vi "Preference_Panel.vi"(0 "Mode":T1) -> ()   [LabVIEW 2010]
uses:
  Anemometry Sub Vis/Controls/Server_Comms.ctl
  Anemometry Sub Vis/Controls/Preference_Mode.ctl
  Anemometry Sub Vis/Controls/Overhead.ctl
  <vilib>/Instr/_visa.llb/VISA Find Search Mode.ctl
  ADAM Client/Sub VIs/ADAM Controls/Calib_type_ADAM.ctl
  ADAM Client/Sub VIs/ADAM Controls/Module_type_ADAM.ctl
  ADAM Client/Sub VIs/ADAM Controls/Ch_description_ADAM.ctl
  ADAM Client/Sub VIs/ADAM Controls/Function_ADAM.ctl
  ADAM Client/Sub VIs/ADAM Controls/Channel_State.ctl
  ADAM Client/Sub VIs/ADAM Controls/Address.ctl
  Anemometry Sub Vis/Globals/Constants_global.vi
  Anemometry Sub Vis/Globals/Preference_global.vi
  Anemometry Sub Vis/Globals/Trav_pos_global.vi
  Anemometry Sub Vis/Globals/Qnet_Globals.vi
  Anemometry Sub Vis/Acquisition/PWA/PWAtasksGLOBAL.vi
  Anemometry Sub Vis/Globals/Dynamic_call_global.ph.vi
panel:
  in  "Post Processing Machine":bool
  in  "Analogue Device Serial No.":string="1188AB4"
  in  "PWA Device Serial No.":string="1187C98"
  in  "ADAM Setup File":u16(ring) items=["Current_Setup.xls"]
  in  "Default Source Establishment Time (s)":dbl=20.0
  out "This Machine's IP Number":string
  in  "Rig Setup":u16(ring) items=["3_x_2_tunnel", "A_Tunnel", "Adam_Sayer_Desk", "ADAM_Server", "Aero_Tunnel", "Alex_Desktop", "B_Tunnel", "Calibration_Tunnel", "Contact_Conductance", "D_Tunnel", "EnFlo_Tunnel", "Frauke_Desktop", "iMac_G5_2", "iMacDuo1", "Matteo's_desktop", "Matteo_PC", "Nick_PC-2", "Paul_Desk-Paul_Desk_Machine", "Paul_Hayden-Desk", "Paul_N_Desk_Machine_2", "Post_Processing_Machine", "PowerBook_G4_1", "PowerBook_G4_2", "Syn_jet_rig", "Tank", "tdf", "Tom_Desk", "Towing_tank", "--New Rig Setup--"]
  in  "Default Traverse Name":u16(ring) items=["A_Tunnel", "Aero_ThroughWall", "Aero_Tunnel", "Angle_Calibrator", "B_Tunnel", "D_Tunnel", "Dummy_Traverse", "EnFlo_Stack", "EnFlo_Tunnel", "EnFlo_Turntable", "Laser_Meas_Traverse", "mohd_setup", "Paul_Desk_Test", "PIV_Traverse", "--New Traverse Setup--"]
  in  "OK":bool
  in  "% Error From First Calib":dbl=10.0 format="%.1f"
  in  "% Error From Previous Calib":dbl=0.5 format="%.1f"
  in  "Qnet Site Root":path=path "/G4_2_HD/Users/paulhayden/Qnet/qnet"
  out "Templates":path=path "/G4_2_HD/Applications (Mac OS 9)/EnFlo Software/Anemometry/Anemometry Sub Vis/Templates"
  in  "Data Folder":path
  out "EnFlo SW Preferences":path=path "/G4_2_HD/Applications (Mac OS 9)/LabVIEW 5.1/EnFlo SW Preferences"
  in  "Tunnel Speed Control":bool
  in  "SMTP server IP address":string
  in  "Abs Press (mbar)":string="Froude:NPL:Atmos_Press"
  in  "Temperature":string="EnFlo Tun:Inlet Heater:Av Temp"
  in  "Server port number":u32=3363
  in  "Server address":string
  in  "LabVIEW Administrators":string[](array[string])=["", "", "", "", "", "", "", "", "", "", "", "", "", "", "", "", "", "", "", ""]
  in  "Server Comms":T2=enum."Do Not Link To Server"
  # "Server Computer Peferences"
  # "Multi Run Preferences"
  # "Warning Levels for Autocalibration Changes"
  # "Email Peferences"
  # "Deg C"
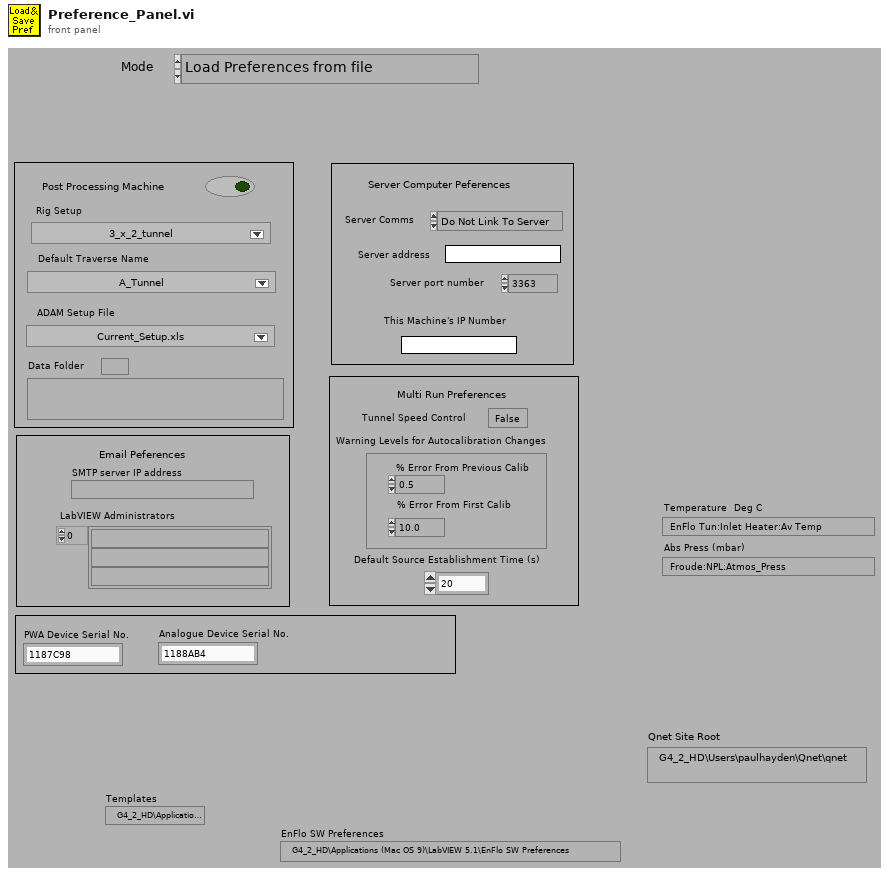
[diagram p1: front panel]
types:
  T1 = typedef "Preference_Mode.ctl" = enum16{"Load Preferences from file", "Save Preferences to file", "Load, Edit then Save"}
  T2 = typedef "Server_Comms.ctl" = enum16{"Server Link Healthy", "Do Not Link To Server"}
  T3 = enum8{"Enabled", "Disabled", "Disabled and Grayed Out"}
  T4 = typedef "Overhead.ctl" = enum16{"Update total times", "Read Current Overhead", "Re Scale totals to 3 hrs", "Initialise totals to 3hr"}
  T5 = typedef "Calib_type_ADAM.ctl" = enum16{"Raw", "Bx + A", "Cx^2 + Bx + A", "Dx^3 + Cx^2 + Bx + A", "In Band", "Hi-Tec Q", "Hi-Tec M_dot", "Text"}
  T6 = typedef "Module_type_ADAM.ctl" = enum16{"4011", "4012", "4013", "4014", "4016", "4017", "4018", "4021", "4050", "4052", "4053", "4060", "4080", "5000", "5017", "5018", "5024", "5051", "5056", "5060", "6060", "Tracker", "WEST", "GILL", "JEM", "VICI", "Vaisala", "DRUCK", "Run VI Named:", "IR2100", "PPT", "Comparator", "VIRTUAL", "Hold Value", "Read A", "Read Ch", "Coded", "Client Info", "Web Client", "X10", "Test"}
  T7 = typedef "Channel_State.ctl" = enum16{"On", "Off", "Always On", "Always Off"}
  T8 = typedef "VISA Find Search Mode.ctl" = u32
  T9 = typedef "Ch_description_ADAM.ctl" = cluster{"Ch Name":string, "Type":T6, "Function":T10, "Ch State":T7, "Calibration type":T5, "A":dbl, "B":dbl, "C":dbl, "D":dbl, "Comments":string, "Address":T11, "String":string, "Duty":u16}
  T10 = typedef "Function_ADAM.ctl" = enum16{"Analogue Input", "Digital Input", "Event counter", "Event rate", "Analogue Output", "Digital Output", "Relay Output"}
  T11 = typedef "Address.ctl" = cluster{"Main":i32, "Ch.":i32, "Sub":i32, "Port Name":string}
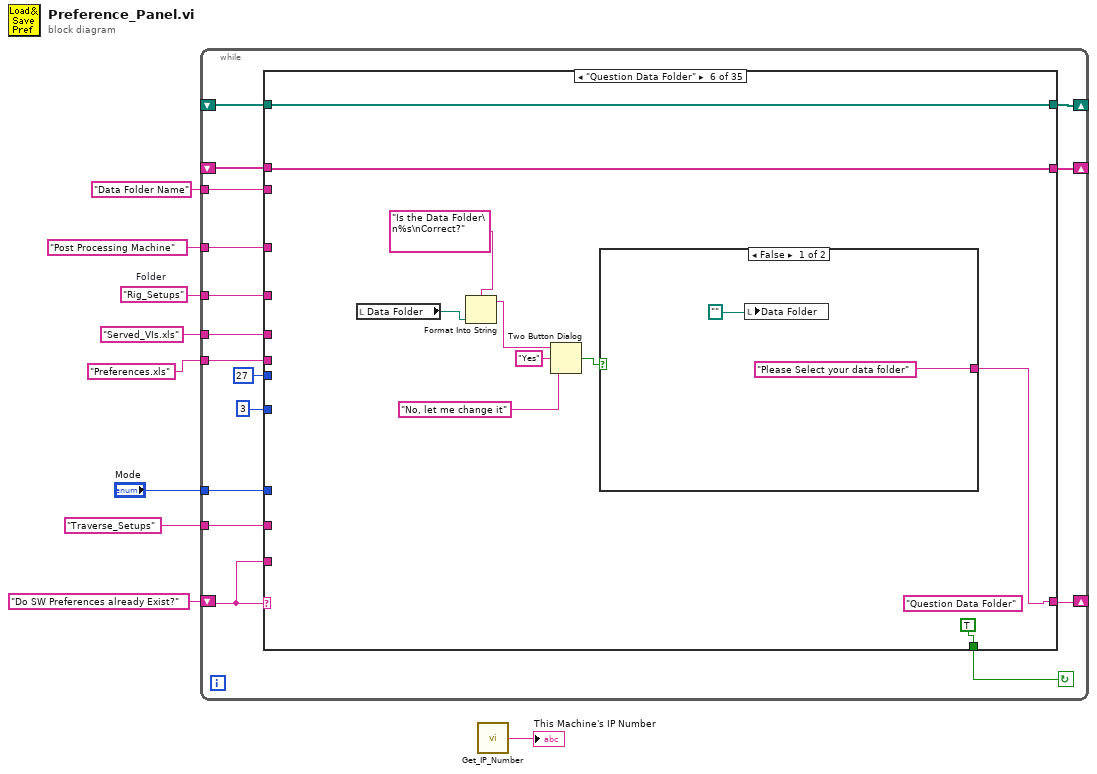
[diagram p0: block diagram]
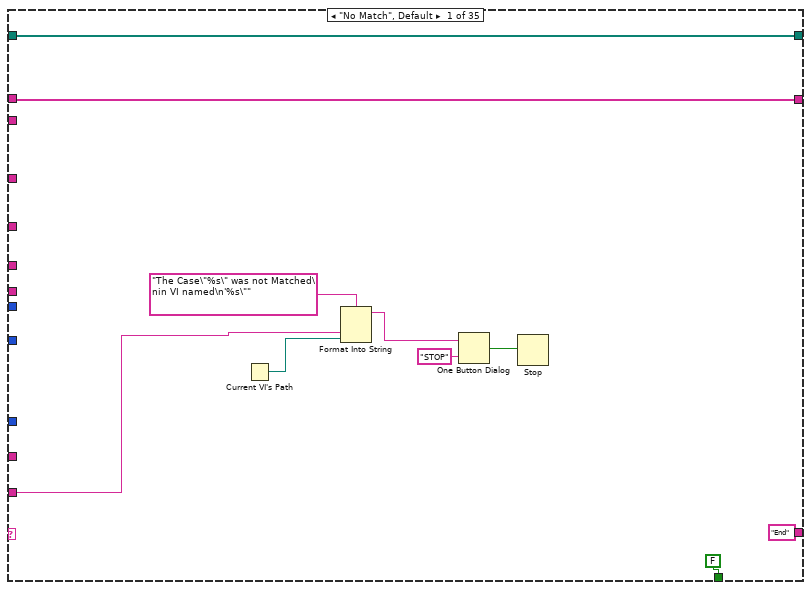
[diagram p2: hidden frame]
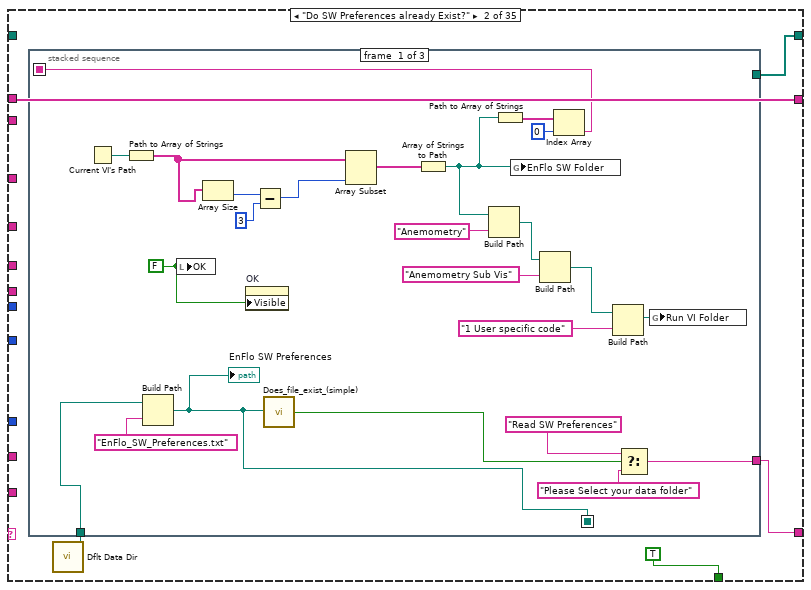
[diagram p3: hidden frame]
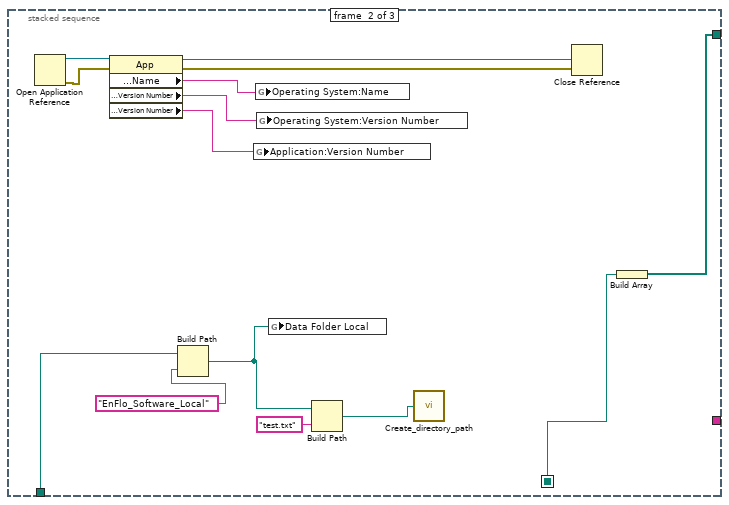
[diagram p4: hidden frame]
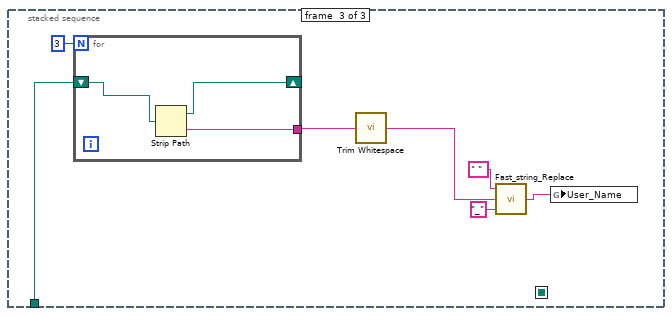
[diagram p5: hidden frame]
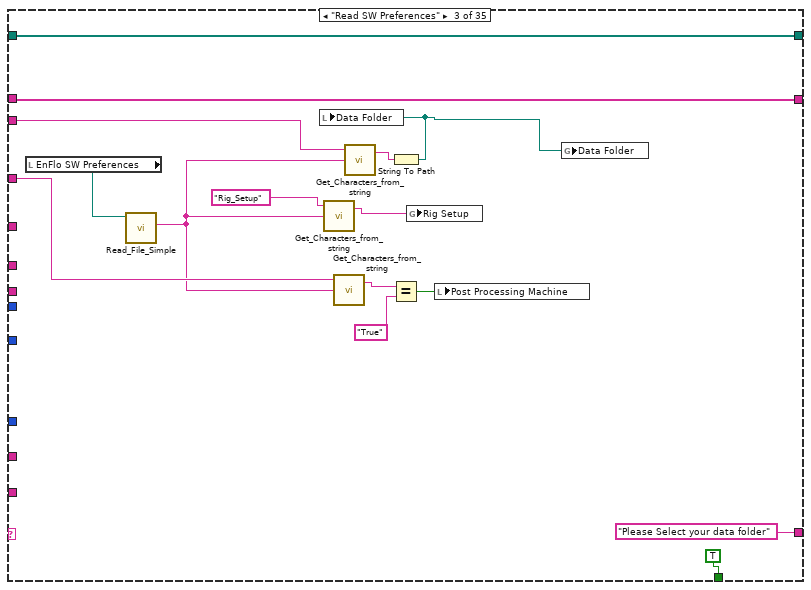
[diagram p6: hidden frame]
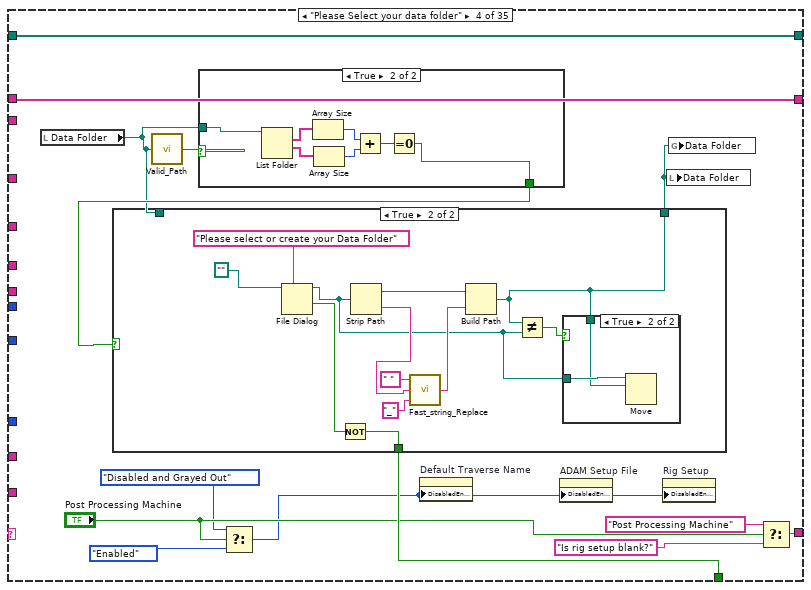
[diagram p7: hidden frame]
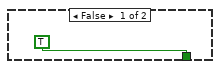
[diagram p8: hidden frame]
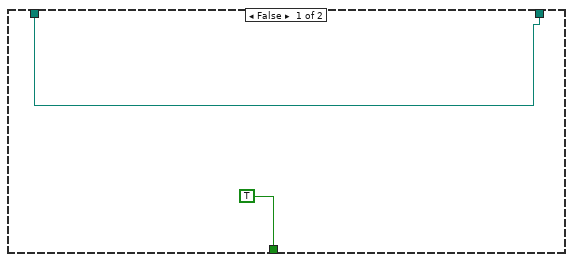
[diagram p9: hidden frame]
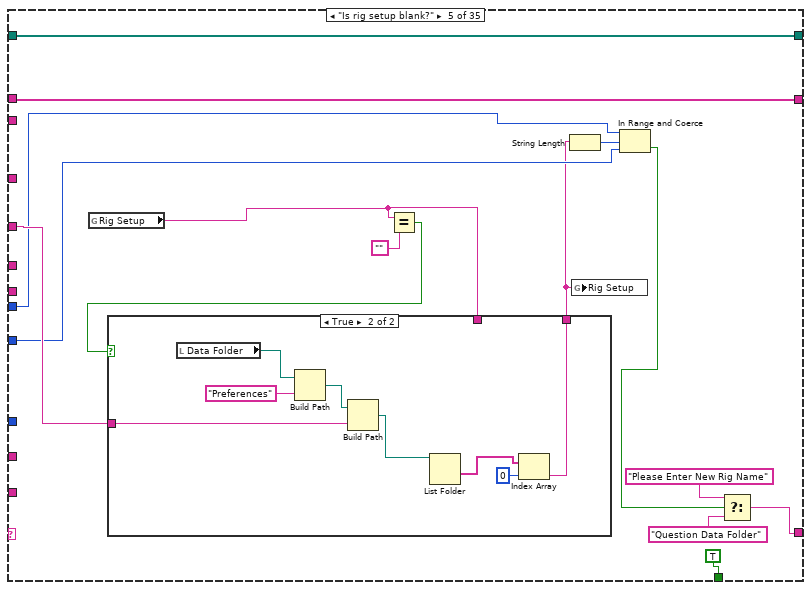
[diagram p11: hidden frame]
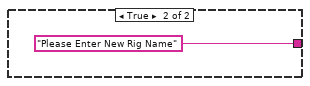
[diagram p13: hidden frame]
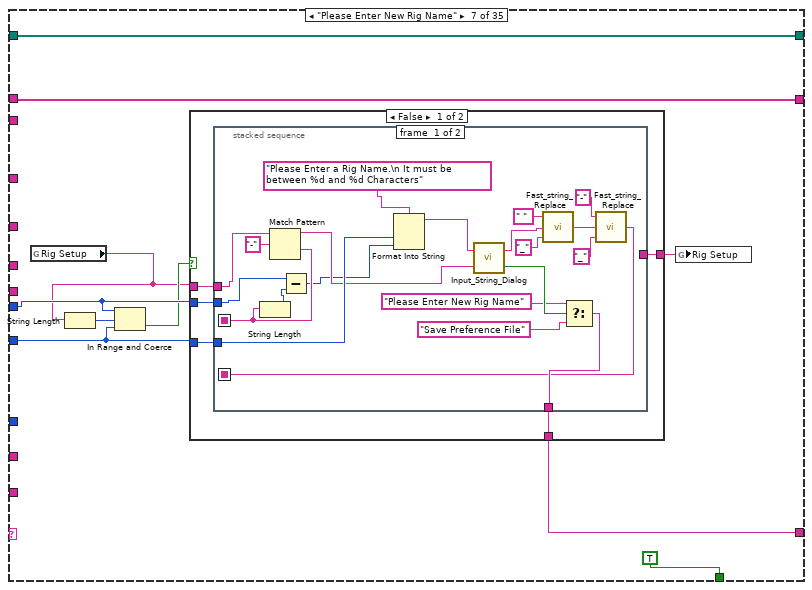
[diagram p14: hidden frame]
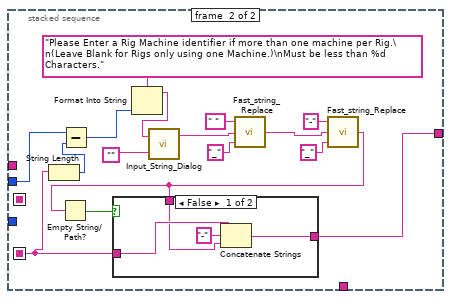
[diagram p15: hidden frame]
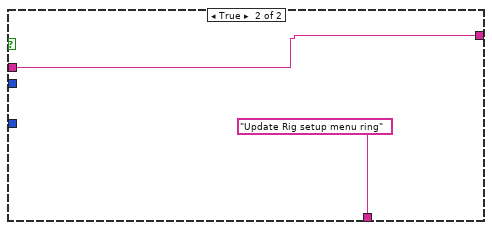
[diagram p17: hidden frame]
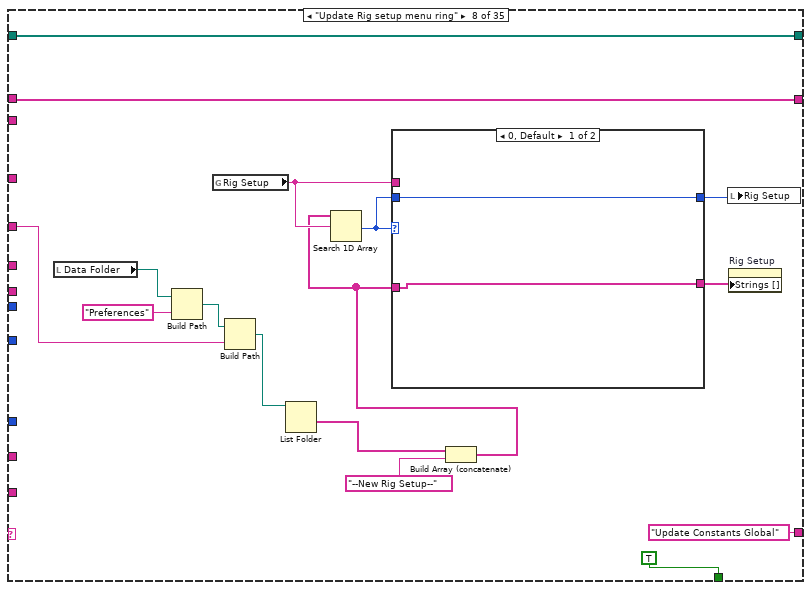
[diagram p18: hidden frame]
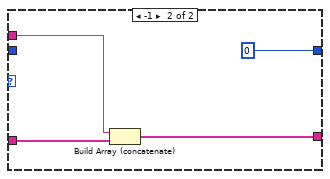
[diagram p19: hidden frame]
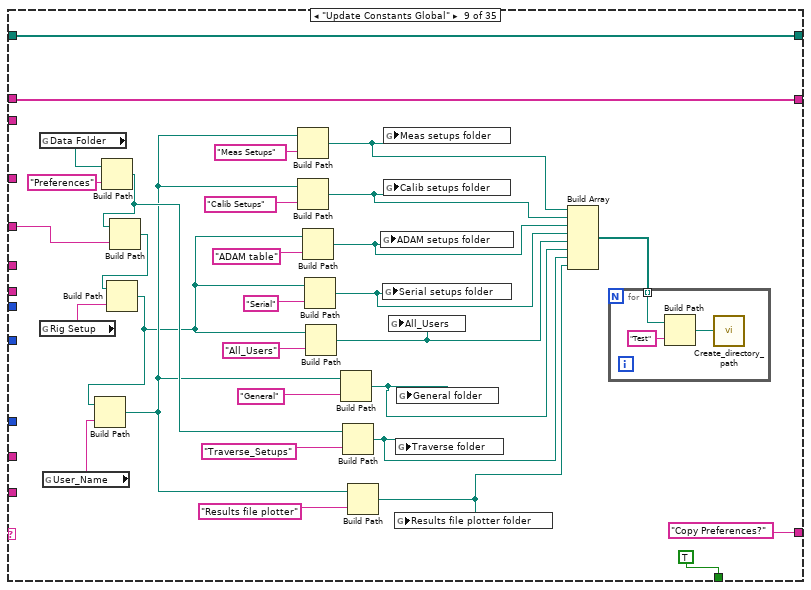
[diagram p20: hidden frame]
diagram:
  w4 = "Rig_Setups"  # Folder
  n1 = while {
    shift-left: _ -> [w22]
    shift-right: [w23] -> _
    shift-left: "Do SW Preferences already Exist?" -> [w21]
    shift-right: [w24] -> _
    tunnel: "Mode" -> [w20]
    tunnel: "Data Folder Name" ("Label for characters") -> [w19]
    tunnel: "Served_VIs.xls" ("Substring") -> [w18]
    tunnel: "Preferences.xls" ("name or relative path") -> [w17]
    tunnel: w4 -> [w14]
    tunnel: "Traverse_Setups" ("name or relative path") -> [w13]
    shift-right: [w12] -> _
    shift-left: _ -> [w11]
    tunnel: "Post Processing Machine" ("Label for characters") -> [w10]
    stop <- w25 continue-if-true
    n2 = case shown="\"Question Data Folder\"" w21 {
      tunnel: [FALSE TRUE TRUE w111 TRUE TRUE TRUE TRUE TRUE TRUE TRUE TRUE TRUE TRUE TRUE TRUE TRUE TRUE TRUE TRUE TRUE TRUE TRUE TRUE TRUE TRUE TRUE TRUE TRUE TRUE w867 TRUE TRUE TRUE FALSE] -> w25
      tunnel: ["End" w38 "Please Select your data folder" w108 w143 w166 w185 "Update Constants Global" ("f") "Copy Preferences?" "Copy Preferences?" w331 "Read SW Preferences" "Install Preference files" "Install Adam table files" "Install Adam setup files" "Choose ADAM Setup file" "Preference files continued" "Variable Names" w506 w523 "Please Enter new  Traverse Setup" w598 "Create Traverse setup" ("f") "Check file permission status" w694 w723 w743 w762 w779 "Save Preference File" "Save SW Preferences" w931 w944 "Initialise Globals" "End"] -> w24
      tunnel: [w27 w39 w102 w117 w155 w174 w187 w252 w288 w321 w329 w345 w392 w408 w433 w452 w474 w485 w511 w533 w586 w600 w634 w651 w695 w728 w748 w771 w784 w798 w873 w939 w945 w997 w1057] -> w23
      tunnel: w22 -> [w27 w39 w102 w117 w155 w174 w187 w252 w288 w321 w329 w345 w392 w408 w433 w452 w474 w485 _ w533 w586 w600 w634 w651 w695 w728 w748 w771 w784 w798 w873 w939 w945 w997 w1057]
      tunnel: w21 -> [w30 _ _ _ _ _ _ _ _ _ _ _ _ _ _ _ _ _ _ _ _ _ _ _ _ _ _ _ _ _ _ _ _ _ _]
      tunnel: w20 -> [_ _ _ _ _ _ _ _ _ _ _ _ _ _ _ _ _ _ w505 _ _ _ _ _ w693 _ _ _ _ _ w868 _ _ _ _]
      tunnel: w19 -> [_ _ w98 _ _ _ _ _ _ _ _ _ _ _ _ _ _ _ _ _ _ _ _ _ _ _ _ _ _ _ _ w930 _ _ _]
      tunnel: w18 -> [_ _ _ _ _ _ _ _ _ _ _ _ _ w402 _ _ _ _ _ _ _ _ _ _ _ _ _ _ _ _ _ _ _ w989 _]
      tunnel: w17 -> [_ _ _ _ _ _ _ _ _ _ w326 w343 _ _ _ _ _ _ _ w529 _ _ _ _ _ _ _ _ _ _ w865 _ _ _ _]
      tunnel: 3 ("lower limit") -> [_ _ _ _ w147 _ w184 _ _ _ _ _ _ _ _ _ _ _ _ _ _ w597 _ _ _ _ _ _ _ _ _ _ _ _ _]
      tunnel: 27 ("upper limit") -> [_ _ _ _ w148 _ w183 _ _ _ _ _ _ _ _ _ _ _ _ _ _ w596 _ _ _ _ _ _ _ _ _ _ _ _ _]
      tunnel: w14 -> [_ _ _ _ w152 _ _ w240 w268 w301 _ w342 _ _ _ _ _ _ _ _ _ _ _ _ _ _ _ _ _ _ _ _ _ _ _]
      tunnel: w13 -> [_ _ _ _ _ _ _ _ _ _ _ _ _ _ _ _ _ _ _ _ w584 _ w621 _ _ _ _ _ _ w797 _ _ _ _ _]
      tunnel: [w26 w36 w94 w112 w150 w173 w179 w238 w265 w300 w330 w346 w383 w398 w426 w449 w460 w476 w498 w527 w583 w592 w620 w647 path[] [] w720 w740 w765 w782 w796 w863 w927 w943 w988 w1054] -> w12
      tunnel: w11 -> [w26 _ w94 w112 w150 w173 w179 w238 w265 w300 w330 w346 w382 w400 w426 w450 w460 w478 w498 w528 w583 w592 w620 w648 w692 w720 w740 w765 w782 w796 w863 w927 w943 w988 w1054]
      tunnel: w10 -> [_ _ w93 _ _ _ _ _ _ _ _ _ _ _ _ _ _ _ _ _ _ _ _ _ _ _ _ _ _ _ _ w921 _ _ _]
      frame "No Match", Default {
        n3 = Current VI's Path() -> (path=w35:path)
        n4 = Format Into String(format string="The Case\"%s\" was not Matched\nin VI named\n'%s\"" ("Format String"), w30, w35) -> (resulting string=w32:string)  [unwired: 2 in, 1 out]
        n5 = One Button Dialog(message=w32, button name ("OK")="STOP") -> (true=w34:bool)
        n6 = Stop(stop? (T)=w34) -> ()
      }
      frame "Do SW Preferences already Exist?" {
        n7 = call <vilib>:"Dflt Data Dir.vi"() -> ("App:Default Data Directory"=w37:path)
        n8 = stacked-sequence {
          seq-local: [w44 _ _] -> [_ _ _]
          seq-local: [w42 _ _] -> [_ w70 _]
          tunnel: [w48 _ _] -> w38
          tunnel: w37 -> [w43 w68 w84]
          tunnel: [_ w71 _] -> w36
          frame #0 {
            w41 = FALSE ("OK")
            n9 = Current VI's Path() -> (path=w62:path)
            n10 = Path to Array of Strings(0:w62) -> (2:w59:string[])  [unwired: 1 out]
            n11 = Build Path(base path=w43, name or relative path="EnFlo_SW_Preferences.txt") -> (appended path=w42:path)
            "EnFlo SW Preferences" <- w42
            n12 = local write "OK"(w41) -> ()
            n13 = Array Size(array=w59) -> (size(s)=w61:i32)
            n14 = property on="OK" class="Bool (strict)"("Visible"=w41) -> ()  [unwired: 2 in, 2 out]
            n15 = Subtract(x=w61, y=3) -> (x-y=w57:i32)
            n16 = call "Does_file_exist_(simple).vi"("Pathname"=w42) -> ("exists?"=w63:bool)
            n17 = Array Subset(array=w59, length=w57) -> (w58:string[])  [unwired: 1 in]
            n18 = Array of Strings to Path(0:w58) -> (2:w45:path)  [unwired: 1 out]
            n19 = Build Path(base path=w45, name or relative path="Anemometry") -> (appended path=w54:path)
            n20 = Path to Array of Strings(0:w45) -> (2:w46:string[])  [unwired: 1 out]
            n21 = global write "Constants_global.vi" "EnFlo SW Folder"(w45) -> ()
            n22 = Build Path(base path=w54, name or relative path="Anemometry Sub Vis") -> (appended path=w52:path)
            n23 = Index Array(array=w46, index=0) -> (element=w44:string)
            n24 = Build Path(base path=w52, name or relative path="1 User specific code") -> (appended path=w51:path)
            n25 = Select(t="Read SW Preferences", s=w63, f="Please Select your data folder") -> (s? t:f=w48:string)
            n26 = global write "Constants_global.vi" "Run VI Folder"(w51) -> ()
          }
          frame #1 {
            n27 = Open Application Reference() -> (0:w75:errorcluster, 3:w78:refnum<vi>)  [unwired: 1 in, 3 out]
            n28 = property class="App"(reference=w78, error in=w75) -> (reference out=w77:refnum<vi>, error out=w76:errorcluster, "Operating System:Name"=w72:string, "Operating System:Version Number"=w74:string, "Application:Version Number"=w73:string)
            n29 = Build Path(base path=w68, name or relative path="EnFlo_Software_Local" ("element")) -> (appended path=w67:path)
            n30 = global write "Preference_global.vi" "Application:Version Number"(w73) -> ()
            n31 = global write "Preference_global.vi" "Operating System:Name"(w72) -> ()
            n32 = global write "Preference_global.vi" "Operating System:Version Number"(w74) -> ()
            n33 = global write "Constants_global.vi" "Data Folder Local"(w67) -> ()
            n34 = Build Path(base path=w67, name or relative path="test.txt") -> (appended path=w65:path)
            n35 = call "Create_directory_path.vi"("Path name"=w65) -> ()  [unwired: 1 out]
            n36 = Close Reference(reference=w77, error in (no error)=w76) -> ()  [unwired: 1 out]
            n37 = Build Array(w70) -> (w71:path[])
          }
          frame #2 {
            n38 = for {
              N: 3 -> [_]
              shift-right: [w88] -> _
              shift-left: w84 -> [w87]
              tunnel: [w86] -> w80
              n39 = Strip Path(path=w87) -> (stripped path=w88:path, name=w86:string)
            }
            n40 = call <vilib>:"Trim Whitespace.vi"("string"=w80) -> ("trimmed string"=w79:string)  [unwired: 1 in]
            n41 = call "Fast_string_Replace.vi"("Replace match with:"="_", "Input String"=w79, "regular expression"=" ") -> ("Output String"=w81:string)  [unwired: 1 in, 1 out]
            n42 = global write "Preference_global.vi" "User_Name"(w81) -> ()
          }
        }
      }
      frame "Read SW Preferences" {
        n43 = local read "EnFlo SW Preferences"() -> (w101:path)
        n44 = call "Read_File_Simple.vi"("Filename"=w101) -> ("string"=w92:string)  [unwired: 2 in, 7 out]
        n45 = call "Get_Characters_from_string.vi"("Input string"=w92, "Variable name"="Rig_Setup" ("Label for characters")) -> ("Value"=w95:string)  [unwired: 1 in, 1 out]
        n46 = call "Get_Characters_from_string.vi"("Input string"=w92, "Variable name"=w93) -> ("Value"=w91:string)  [unwired: 1 in, 1 out]
        n47 = call "Get_Characters_from_string.vi"("Input string"=w92, "Variable name"=w98) -> ("Value"=w99:string)  [unwired: 1 in, 1 out]
        n48 = String To Path(string=w99) -> (path=w97:path)
        n49 = local write "Data Folder"(w97) -> ()
        n50 = Equal?(x=w91, y="True") -> (x = y?=w89:bool)
        n51 = global write "Preference_global.vi" "Rig Setup"(w95) -> ()
        n52 = local write "Post Processing Machine"(w89) -> ()
        n53 = global write "Constants_global.vi" "Data Folder"(w97) -> ()
      }
      frame "Please Select your data folder" {
        n54 = local read "Data Folder"() -> (w113:path)
        n55 = call "Valid_Path.vi"("Filename"=w113) -> ("Valid Path?"=w115:bool)
        n56 = case shown="True" w115 {
          tunnel: [TRUE ("status") w119] -> w114
          tunnel: w113 -> [_ w125]
          frame False {
          }
          frame True {
            n57 = List Folder(path=w125) -> (filenames=w123:string[], folder names=w124:string[])  [unwired: 1 in, 4 out]
            n58 = Array Size(array=w123) -> (size(s)=w121:i32)
            n59 = Array Size(array=w124) -> (size(s)=w122:i32)
            n60 = Add(x=w121, y=w122) -> (x+y=w120:i32)
            n61 = Equal To 0?(x=w120) -> (x = 0?=w119:bool)
          }
        }
        n62 = case shown="True" w114 {
          tunnel: [w127 w130] -> w116
          tunnel: w113 -> [w127 _]
          tunnel: [TRUE w128] -> w111
          frame False {
          }
          frame True {
            n63 = File Dialog(7:"Please select or create your Data Folder" ("prompt"), 11:path "") -> (1:w129:bool, 3:w131:path)  [unwired: 1 in, 6 out]
            n64 = Not(x=w129) -> (.not. x?=w128:bool)
            n65 = Strip Path(path=w131) -> (stripped path=w135:path, name=w134:string)
            n66 = call "Fast_string_Replace.vi"("Replace match with:"="_", "Input String"=w134, "regular expression"=" ") -> ("Output String"=w133:string)  [unwired: 2 out]
            n67 = Build Path(base path=w135, name or relative path=w133) -> (appended path=w130:path)
            n68 = Not Equal?(x=w130, y=w131) -> (x != y?=w132:bool)
            n69 = case shown="True" w132 {
              tunnel: w131 -> [_ w141]
              tunnel: w130 -> [_ w140]
              frame False {
              }
              frame True {
                n70 = Move(source path=w141, 10:w140) -> ()  [unwired: 1 in, 5 out]
              }
            }
          }
        }
        n71 = Select(t=T3."Disabled and Grayed Out" ("Disabled"), s="Post Processing Machine", f=T3."Enabled" ("Disabled")) -> (s? t:f=w104:T3)
        n72 = property on="Default Traverse Name" class="Ring (strict)"("DisabledEnum"=w104) -> ()  [unwired: 2 in, 2 out]
        n73 = property on="ADAM Setup File" class="Ring (strict)"("DisabledEnum"=w104) -> ()  [unwired: 2 in, 2 out]
        n74 = property on="Rig Setup" class="Ring (strict)"("DisabledEnum"=w104) -> ()  [unwired: 2 in, 2 out]
        n75 = local write "Data Folder"(w116) -> ()
        n76 = global write "Constants_global.vi" "Data Folder"(w116) -> ()
        n77 = Select(t="Post Processing Machine", s="Post Processing Machine", f="Is rig setup blank?") -> (s? t:f=w108:string)
      }
      frame "Is rig setup blank?" {
        n78 = global read "Preference_global.vi" "Rig Setup"() -> (w151:string)
        n79 = Equal?(x=w151, y="") -> (x = y?=w153:bool)
        n80 = case shown="True" w153 {
          tunnel: w152 -> [_ w161]
          tunnel: [w157 w158] -> w146
          tunnel: w151 -> [w157 _]
          frame False {
          }
          frame True {
            n81 = local read "Data Folder"() -> (w164:path)
            n82 = Build Path(base path=w164, name or relative path="Preferences") -> (appended path=w163:path)
            n83 = Build Path(base path=w163, name or relative path=w161) -> (appended path=w162:path)
            n84 = List Folder(path=w162) -> (folder names=w159:string[])  [unwired: 1 in, 5 out]
            n85 = Index Array(array=w159, index=0) -> (element=w158:string)
          }
        }
        n86 = String Length(string=w146) -> (length=w149:i32)
        n87 = global write "Preference_global.vi" "Rig Setup"(w146) -> ()
        n88 = In Range and Coerce(upper limit=w148, x=w149, lower limit=w147) -> (In Range?=w145:bool)  [unwired: 1 out]
        n89 = Select(t="Please Enter New Rig Name", s=w145, f="Question Data Folder") -> (s? t:f=w143:string)
      }
      frame "Question Data Folder" {
        (unwired) "Question Data Folder"
        n90 = local read "Data Folder"() -> (w172:path)
        n91 = Format Into String(format string="Is the Data Folder\n%s\nCorrect?" ("message"), w172) -> (resulting string=w170:string)  [unwired: 2 in, 1 out]
        n92 = Two Button Dialog(message=w170, 1:"No, let me change it" ("F button name (\"Cancel\")"), 2:"Yes" ("T button name (\"OK\")")) -> (T button?=w167:bool)
        n93 = case shown="False" w167 {
          tunnel: ["Please Select your data folder" "Please Enter New Rig Name"] -> w166
          frame False {
            n94 = local write "Data Folder"(path "") -> ()
          }
          frame True {
          }
        }
      }
      frame "Please Enter New Rig Name" {
        n95 = global read "Preference_global.vi" "Rig Setup"() -> (w181:string)
        n96 = String Length(string=w181) -> (length=w186:i32)
        n97 = In Range and Coerce(upper limit=w183, x=w186, lower limit=w184) -> (In Range?=w182:bool)  [unwired: 1 out]
        n98 = case shown="False" w182 {
          tunnel: w181 -> [w193 w236]
          tunnel: [w189 "Update Rig setup menu ring"] -> w185
          tunnel: [w190 w236] -> w180
          tunnel: w184 -> [w192 _]
          tunnel: w183 -> [w191 _]
          frame False {
            n99 = stacked-sequence {
              seq-local: [w194 _] -> [_ w219]
              seq-local: [w201 _] -> [_ _]
              tunnel: w193 -> [w203 _]
              tunnel: w192 -> [w214 _]
              tunnel: w191 -> [w200 w217]
              tunnel: [_ w222] -> w190
              tunnel: [w206 _] -> w189
              frame #0 {
                n100 = Match Pattern(string=w203, regular expression="-") -> (before substring=w202:string, after substring=w201:string)  [unwired: 3 out]
                n101 = String Length(string=w201) -> (length=w199:i32)
                n102 = Subtract(x=w200, y=w199) -> (x-y=w198:i32)
                n103 = Format Into String(format string="Please Enter a Rig Name.\n It must be between %d and %d Characters" ("Message to user"), w214, w198) -> (resulting string=w213:string)  [unwired: 2 in, 1 out]
                n104 = call "Input_String_Dialog.vi"("Value"=w202, "Message to user"=w213) -> ("Ok Out"=w209:bool, "Output string"=w210:string)
                n105 = call "Fast_string_Replace.vi"("Replace match with:"="_", "Input String"=w210, "regular expression"=" ") -> ("Output String"=w195:string)  [unwired: 2 out]
                n106 = Select(t="Please Enter New Rig Name", s=w209, f="Save Preference File") -> (s? t:f=w206:string)
                n107 = call "Fast_string_Replace.vi"("Replace match with:"="_", "Input String"=w195, "regular expression"="-") -> ("Output String"=w194:string)  [unwired: 2 out]
              }
              frame #1 {
                n108 = String Length(string=w219) -> (length=w218:i32)
                n109 = Subtract(x=w217, y=w218) -> (x-y=w216:i32)
                n110 = Format Into String(format string="Please Enter a Rig Machine identifier if more than one machine per Rig.\n(Leave Blank for Rigs only using one Machine.)\nMust be less than %d Characters." ("Message to user"), w216) -> (resulting string=w215:string)  [unwired: 2 in, 1 out]
                n111 = call "Input_String_Dialog.vi"("Value"="", "Message to user"=w215) -> ("Output string"=w228:string)  [unwired: 1 out]
                n112 = call "Fast_string_Replace.vi"("Replace match with:"="_", "Input String"=w228, "regular expression"=" ") -> ("Output String"=w224:string)  [unwired: 2 out]
                n113 = call "Fast_string_Replace.vi"("Replace match with:"="_", "Input String"=w224, "regular expression"="-") -> ("Output String"=w221:string)  [unwired: 2 out]
                n114 = Empty String/Path?(string/path=w221) -> (empty?=w223:bool)
                n115 = case shown="False" w223 {
                  tunnel: [w231 w235] -> w222
                  tunnel: w219 -> [w234 w235]
                  tunnel: w221 -> [w232 _]
                  frame False {
                    n116 = Concatenate Strings(w234, "-" ("string"), w232) -> (w231:string)
                  }
                  frame True {
                  }
                }
              }
            }
          }
          frame True {
          }
        }
        n117 = global write "Preference_global.vi" "Rig Setup"(w180) -> ()
      }
      frame "Update Rig setup menu ring" {
        n118 = local read "Data Folder"() -> (w243:path)
        n119 = Build Path(base path=w243, name or relative path="Preferences") -> (appended path=w242:path)
        n120 = global read "Preference_global.vi" "Rig Setup"() -> (w249:string)
        n121 = Build Path(base path=w242, name or relative path=w240) -> (appended path=w241:path)
        n122 = List Folder(path=w241) -> (folder names=w239:string[])  [unwired: 1 in, 5 out]
        n123 = Build Array (concatenate)(w239, "--New Rig Setup--") -> (w245:string[])
        n124 = Search 1D Array(1D array=w245, element=w249) -> (index of element=w248:i32)  [unwired: 1 out]
        n125 = case shown="0, Default" w248 {
          tunnel: [w255 0] -> w251
          tunnel: w245 -> [w254 w258]
          tunnel: w249 -> [_ w257]
          tunnel: w248 -> [w255 _]
          tunnel: [w254 w256] -> w247
          frame 0, Default {
          }
          frame -1 {
            n126 = Build Array (concatenate)(w257, w258) -> (w256:string[])
          }
        }
        n127 = local write "Rig Setup"(w251) -> ()
        n128 = property on="Rig Setup" class="Ring (strict)"("Strings []"=w247) -> ()  [unwired: 2 in, 2 out]
      }
      frame "Update Constants Global" {
        n129 = global read "Constants_global.vi" "Data Folder"() -> (w266:path)
        n130 = global read "Preference_global.vi" "Rig Setup"() -> (w267:string)
        n131 = global read "Preference_global.vi" "User_Name"() -> (w264:string)
        n132 = Build Path(base path=w266, name or relative path="Preferences") -> (appended path=w269:path)
        n133 = Build Path(base path=w269, name or relative path=w268) -> (appended path=w270:path)
        n134 = Build Path(base path=w270, name or relative path=w267) -> (appended path=w260:path)
        n135 = Build Path(base path=w260, name or relative path=w264) -> (appended path=w263:path)
        n136 = Build Path(base path=w263, name or relative path="Meas Setups") -> (appended path=w280:path)
        n137 = Build Path(base path=w263, name or relative path="Calib Setups") -> (appended path=w279:path)
        n138 = Build Path(base path=w260, name or relative path="ADAM table") -> (appended path=w278:path)
        n139 = Build Path(base path=w260, name or relative path="Serial") -> (appended path=w277:path)
        n140 = Build Path(base path=w260, name or relative path="All_Users") -> (appended path=w261:path)
        n141 = Build Path(base path=w263, name or relative path="General") -> (appended path=w276:path)
        n142 = Build Path(base path=w269, name or relative path="Traverse_Setups") -> (appended path=w275:path)
        n143 = Build Path(base path=w263, name or relative path="Results file plotter") -> (appended path=w271:path)
        n144 = global write "Constants_global.vi" "ADAM setups folder"(w278) -> ()
        n145 = global write "Constants_global.vi" "Serial setups folder"(w277) -> ()
        n146 = global write "Constants_global.vi" "Meas setups folder"(w280) -> ()
        n147 = global write "Constants_global.vi" "Calib setups folder"(w279) -> ()
        n148 = global write "Constants_global.vi" "All_Users"(w261) -> ()
        n149 = global write "Constants_global.vi" "Results file plotter folder"(w271) -> ()
        n150 = global write "Constants_global.vi" "Traverse folder"(w275) -> ()
        n151 = global write "Constants_global.vi" "General folder"(w276) -> ()
        n152 = Build Array(w280, w279, w278, w277, w261, w276, w275, w271) -> (w274:path[])
        n153 = for {
          tunnel: w274 -> [w292] mode=indexing
          n154 = Build Path(base path=w292, name or relative path="Test") -> (appended path=w290:path)
          n155 = call "Create_directory_path.vi"("Path name"=w290) -> ()  [unwired: 1 out]
        }
      }
      frame "Post Processing Machine" {
        w298 = "Post_Processing_Machine" ("Rig Setup")
        n156 = global read "Constants_global.vi" "Data Folder Local"() -> (w299:path)
        n157 = global read "Preference_global.vi" "User_Name"() -> (w297:string)
        n158 = global write "Preference_global.vi" "Rig Setup"(w298) -> ()
        n159 = Build Path(base path=w299, name or relative path="Preferences") -> (appended path=w302:path)
        n160 = Build Path(base path=w302, name or relative path=w301) -> (appended path=w303:path)
        n161 = Build Path(base path=w303, name or relative path=w298) -> (appended path=w293:path)
        n162 = Build Path(base path=w293, name or relative path=w297) -> (appended path=w296:path)
        n163 = Build Path(base path=w296, name or relative path="Meas Setups") -> (appended path=w313:path)
        n164 = Build Path(base path=w296, name or relative path="Calib Setups") -> (appended path=w312:path)
        n165 = Build Path(base path=w293, name or relative path="ADAM table") -> (appended path=w311:path)
        n166 = Build Path(base path=w293, name or relative path="Serial") -> (appended path=w310:path)
        n167 = Build Path(base path=w293, name or relative path="All_Users") -> (appended path=w294:path)
        n168 = Build Path(base path=w296, name or relative path="General") -> (appended path=w309:path)
        n169 = Build Path(base path=w302, name or relative path="Traverse_Setups") -> (appended path=w308:path)
        n170 = Build Path(base path=w296, name or relative path="Results file plotter") -> (appended path=w304:path)
        n171 = global write "Constants_global.vi" "ADAM setups folder"(w311) -> ()
        n172 = global write "Constants_global.vi" "Serial setups folder"(w310) -> ()
        n173 = global write "Constants_global.vi" "Meas setups folder"(w313) -> ()
        n174 = global write "Constants_global.vi" "Calib setups folder"(w312) -> ()
        n175 = global write "Constants_global.vi" "All_Users"(w294) -> ()
        n176 = global write "Constants_global.vi" "Results file plotter folder"(w304) -> ()
        n177 = global write "Constants_global.vi" "Traverse folder"(w308) -> ()
        n178 = global write "Constants_global.vi" "General folder"(w309) -> ()
        n179 = Build Array(w313, w312, w311, w310, w294, w309, w308, w304) -> (w307:path[])
        n180 = for {
          tunnel: w307 -> [w325] mode=indexing
          n181 = Build Path(base path=w325, name or relative path="Test") -> (appended path=w323:path)
          n182 = call "Create_directory_path.vi"("Path name"=w323) -> ()  [unwired: 1 out]
        }
      }
      frame "Copy Preferences?" {
        n183 = global read "Constants_global.vi" "General folder"() -> (w336:path)
        n184 = Build Path(base path=w336, name or relative path=w326) -> (appended path=w335:path)
        n185 = call <vilib>:"Check if File or Folder Exists.vi"("path"=w335) -> ("file or folder exists?"=w328:bool)  [unwired: 1 in, 9 out]
        n186 = case shown="False" w328 {
          tunnel: [w337 TRUE ("Error?")] -> w327
          frame False {
            n187 = global read "Constants_global.vi" "All_Users"() -> (w339:path)
            n188 = Build Path(base path=w339, name or relative path="Current_Username") -> (appended path=w340:path)
            n189 = call "Read_File_Simple.vi"("Filename"=w340) -> ("Error?"=w337:bool)  [unwired: 4 in, 5 out]
          }
          frame True {
          }
        }
        n190 = Select(t="Install Generic Meas Setup file", s=w327, f="Copy from last user") -> (s? t:f=w331:string)
      }
      frame "Copy from last user" {
        n191 = stacked-sequence {
          seq-local: [w352 _ _ _] -> [_ w361 w367 w374]
          tunnel: w343 -> [_ w360 _ _]
          tunnel: w342 -> [w348 _ _ _]
          frame #0 {
            n192 = global read "Constants_global.vi" "All_Users"() -> (w357:path)
            n193 = global read "Constants_global.vi" "Data Folder"() -> (w351:path)
            n194 = Build Path(base path=w357, name or relative path="Current_Username") -> (appended path=w355:path)
            n195 = global read "Preference_global.vi" "Rig Setup"() -> (w359:string)
            n196 = call "Read_File_Simple.vi"("Filename"=w355) -> ("string"=w354:string)  [unwired: 4 in, 5 out]
            n197 = Build Path(base path=w351, name or relative path="Preferences") -> (appended path=w350:path)
            n198 = Build Path(base path=w350, name or relative path=w348) -> (appended path=w349:path)
            n199 = Build Path(base path=w349, name or relative path=w359) -> (appended path=w353:path)
            n200 = Build Path(base path=w353, name or relative path=w354) -> (appended path=w352:path)
          }
          frame #1 {
            n201 = global read "Constants_global.vi" "General folder"() -> (w363:path)
            n202 = Build Path(base path=w363, name or relative path=w360) -> (appended path=w362:path)
            n203 = Build Path(base path=w361, name or relative path="General") -> (appended path=w365:path)
            n204 = Build Path(base path=w365, name or relative path=w360) -> (appended path=w364:path)
            n205 = Copy(10:w362, 11:w364) -> ()  [unwired: 3 in, 3 out]
          }
          frame #2 {
            w370 = "Current_Setup.xls"
            n206 = Build Path(base path=w367, name or relative path="Meas Setups") -> (appended path=w371:path)
            n207 = global read "Constants_global.vi" "Meas setups folder"() -> (w372:path)
            n208 = Build Path(base path=w371, name or relative path=w370) -> (appended path=w369:path)
            n209 = Build Path(base path=w372, name or relative path=w370) -> (appended path=w368:path)
            n210 = Copy(10:w368, 11:w369) -> ()  [unwired: 3 in, 3 out]
          }
          frame #3 {
            w377 = "Current_Setup.xls"
            n211 = Build Path(base path=w374, name or relative path="Calib Setups") -> (appended path=w378:path)
            n212 = global read "Constants_global.vi" "Calib setups folder"() -> (w379:path)
            n213 = Build Path(base path=w378, name or relative path=w377) -> (appended path=w376:path)
            n214 = Build Path(base path=w379, name or relative path=w377) -> (appended path=w375:path)
            n215 = Copy(10:w375, 11:w376) -> ()  [unwired: 3 in, 3 out]
          }
        }
      }
      frame "Install Generic Meas Setup file" {
        n216 = global read "Constants_global.vi" "Run VI Folder"() -> (w391:path)
        n217 = global read "Constants_global.vi" "Meas setups folder"() -> (w388:path)
        n218 = Strip Path(path=w391) -> (stripped path=w389:path)  [unwired: 1 out]
        n219 = Build Path(base path=w388, name or relative path="Current_Setup.xls") -> (appended path=w381:path)
        n220 = Build Path(base path=w389, name or relative path="Templates") -> (appended path=w385:path)
        "Templates" <- w385
        n221 = call "Does_file_exist_(simple).vi"("Pathname"=w381) -> ("exists?"=w386:bool)
        n222 = case shown="False" w386 {
          tunnel: w381 -> [w397 _]
          tunnel: w385 -> [w395 _]
          frame False {
            n223 = Build Path(base path=w395, name or relative path="Measurement Setup.xls") -> (appended path=w394:path)
            n224 = Copy(10:w397, 11:w394) -> ()  [unwired: 1 in, 5 out]
          }
          frame True {
          }
        }
        n225 = Build Array (concatenate)(w382, w381) -> (w383:path[])
      }
      frame "Install Preference files" {
        n226 = global read "Constants_global.vi" "General folder"() -> (w405:path)
        n227 = Build Array("Preferences.xls" ("Substring"), w402, "Month_Names.xls" ("name or relative path"), "LDA_Configuration.xls") -> (w407:string[])
        n228 = for {
          tunnel: w407 -> [w411] mode=indexing
          tunnel: w405 -> [w412]
          tunnel: [w410] -> w399 mode=indexing
          n229 = Build Path(base path=w412, name or relative path=w411) -> (appended path=w410:path)
          n230 = call "Does_file_exist_(simple).vi"("Pathname"=w410) -> ("exists?"=w413:bool)
          n231 = case shown="False" w413 {
            tunnel: w410 -> [w417 _]
            tunnel: w411 -> [w414 _]
            frame False {
              n232 = local read "Templates"() -> (w415:path)
              n233 = Build Path(base path=w415, name or relative path=w414) -> (appended path=w416:path)
              n234 = Copy(10:w417, 11:w416) -> ()  [unwired: 1 in, 5 out]
            }
            frame True {
            }
          }
        }
        n235 = Build Array (concatenate)(w400, w399) -> (w398:path[])
      }
      frame "Install Adam table files" {
        w422 = "Current_Setup.xls"
        n236 = global read "Constants_global.vi" "ADAM setups folder"() -> (w424:path)
        n237 = Build Path(base path=w424, name or relative path=w422) -> (appended path=w425:path)
        n238 = Build Path(base path=w424, name or relative path="Setup_Files") -> (appended path=w420:path)
        n239 = Build Array("Hi_Tec_Calibs.xls" ("name or relative path"), "A_Tunnel DB setup.xls" ("Substring"), "EnFlo_Tunnel DB setup.xls", "Aero_Tunnel DB setup.xls" ("name or relative path"), "D_Tunnel DB setup.xls") -> (w432:string[])
        n240 = Build Path(base path=w420, name or relative path=w422) -> (appended path=w419:path)
        n241 = for {
          tunnel: w432 -> [w436] mode=indexing
          tunnel: w424 -> [w437]
          n242 = Build Path(base path=w437, name or relative path=w436) -> (appended path=w435:path)
          n243 = call "Does_file_exist_(simple).vi"("Pathname"=w435) -> ("exists?"=w438:bool)
          n244 = case shown="False" w438 {
            tunnel: w435 -> [w442 _]
            tunnel: w436 -> [w439 _]
            frame False {
              n245 = local read "Templates"() -> (w440:path)
              n246 = Build Path(base path=w440, name or relative path=w439) -> (appended path=w441:path)
              n247 = Copy(10:w442, 11:w441) -> ()  [unwired: 1 in, 5 out]
            }
            frame True {
            }
          }
        }
        n248 = call "Create_directory_path.vi"("Path name"=w419) -> ("Path name Out"=w418:path)
        n249 = Move(source path=w425, 10:w418) -> ()  [unwired: 1 in, 5 out]
      }
      frame "Install Adam setup files" {
        w446 = "Current_Setup.xls"
        n250 = global read "Constants_global.vi" "ADAM setups folder"() -> (w448:path)
        n251 = Build Path(base path=w448, name or relative path="Setup_Files") -> (appended path=w445:path)
        n252 = Build Path(base path=w445, name or relative path=w446) -> (appended path=w443:path)
        n253 = call "Does_file_exist_(simple).vi"("Pathname"=w443) -> ("exists?"=w444:bool)
        n254 = case shown="False" w444 {
          tunnel: w443 -> [w459 _]
          tunnel: w446 -> [w457 _]
          frame False {
            n255 = local read "Templates"() -> (w458:path)
            n256 = Build Path(base path=w458, name or relative path="ADAM_Setup_files") -> (appended path=w456:path)
            n257 = Build Path(base path=w456, name or relative path=w457) -> (appended path=w455:path)
            n258 = Copy(10:w459, 11:w455) -> ()  [unwired: 1 in, 5 out]
          }
          frame True {
          }
        }
        n259 = Build Array (concatenate)(w450, w443) -> (w449:path[])
      }
      frame "Choose ADAM Setup file" {
        w468 = "Selected_Filename.txt" ("Substring")
        n260 = global read "Constants_global.vi" "ADAM setups folder"() -> (w472:path)
        n261 = Build Path(base path=w472, name or relative path="Setup_Files") -> (appended path=w469:path)
        n262 = Build Path(base path=w469, name or relative path=w468) -> (appended path=w467:path)
        n263 = call "Read_File_Simple.vi"("Filename"=w467) -> ("string"=w465:string)  [unwired: 2 in, 7 out]
        n264 = Build Array(w468) -> (w470:string[])
        n265 = call "List_files_in_order_of_age.vi"("Files to Hide"=w470, "Folder"=w469) -> ("file names"=w466:string[])
        n266 = Search 1D Array(1D array=w466, element=w465) -> (index of element=w462:i32)  [unwired: 1 out]
        n267 = property on="ADAM Setup File" class="Ring (strict)"("Strings []"=w466) -> ()  [unwired: 2 in, 2 out]
        n268 = Less Than 0?(x=w462) -> (x < 0?=w463:bool)
        n269 = Select(t=0, s=w463, f=w462) -> (s? t:f=w461:i32)
        n270 = local write "ADAM Setup File"(w461) -> ()
      }
      frame "Preference files continued" {
        n271 = global read "Constants_global.vi" "Calib setups folder"() -> (w484:path)
        n272 = Build Array("Hot_Wire_Bridges.txt", "Hot_Wire_Probes.txt", "Pressure_Transducers.txt") -> (w479:string[])
        n273 = for {
          tunnel: w479 -> [w488] mode=indexing
          tunnel: w484 -> [w489]
          tunnel: [w487] -> w477 mode=indexing
          n274 = Build Path(base path=w489, name or relative path=w488) -> (appended path=w487:path)
          n275 = call "Does_file_exist_(simple).vi"("Pathname"=w487) -> ("exists?"=w490:bool)
          n276 = case shown="False" w490 {
            tunnel: w487 -> [w494 _]
            tunnel: w488 -> [w491 _]
            frame False {
              n277 = local read "Templates"() -> (w492:path)
              n278 = Build Path(base path=w492, name or relative path=w491) -> (appended path=w493:path)
              n279 = Copy(10:w494, 11:w493) -> ()  [unwired: 1 in, 5 out]
            }
            frame True {
            }
          }
        }
        n280 = Build Array (concatenate)(w478, w477) -> (w476:path[])
      }
      frame "Variable Names" {
        n281 = Build Array("PWA Device Serial No.", "Analogue Device Serial No.", "Server address", "Server port number", "LabVIEW Administrators", "SMTP server IP address", "Server Comms", "Default Source Establishment Time (s)", "Temperature", "Abs Press (mbar)", "Default Traverse Name", "Tunnel Speed Control", "Current Overhead Factor", "Qnet Site Root", "Auto Calib Error fr Previous", "Auto Calib Error fr First") -> (w511:string[])
        n282 = case shown="\"Load, Edit then Save\"" w505 {
          tunnel: ["Load From Preference file" w517 "Save Preference File"] -> w506
          frame "Load Preferences from file" {
          }
          frame "Load, Edit then Save" {
            n283 = local read "OK"() -> (w520:bool)
            n284 = Select(t="Save Preference File", s=w520, f="Load From Preference file") -> (s? t:f=w517:string)
          }
          frame "Save Preferences to file" {
          }
        }
      }
      frame "Load From Preference file" {
        n285 = global read "Constants_global.vi" "General folder"() -> (w530:path)
        n286 = Build Path(base path=w530, name or relative path=w529) -> (appended path=w526:path)
        n287 = call "Read_File_Simple.vi"("Filename"=w526) -> ("string"=w531:string)  [unwired: 2 in, 7 out]
        n288 = for {
          tunnel: w533 -> [w536] mode=indexing
          tunnel: w531 -> [w535]
          w538 = FALSE  # Show Dialog?
          n289 = call "Get_Characters_from_string.vi"("Show Dialog?"=w538, "Input string"=w535, "Variable name"=w536) -> ("Status"=w537:enum16{"Char in string", "Char not in string"}, "Value"=w534:string)
          n290 = case shown="\"Char in string\"" w537 {
            tunnel: w536 -> [w540 _]
            tunnel: w534 -> [w539 _]
            frame "Char in string" {
              n291 = case shown="\"Server address\"" w540 {
                tunnel: w540 -> [w542 _ _ _ _ _ _ _ _ _ _ _ _ _ _ _ _]
                tunnel: w539 -> [_ w543 w544 w547 w548 w549 w551 w553 w556 _ w560 w564 w565 w567 w569 w572 w574]
                tunnel: w539 -> [_ _ _ _ _ _ _ _ _ w557 _ _ _ _ _ _ _]
                frame "No Match", Default {
                  n292 = call "Was_string_matched.vi"("Match Error"=TRUE, "Variable name"=w542) -> ()  [unwired: 1 in]
                }
                frame "Server address" {
                  n293 = global write "Preference_global.vi" "Server address"(w543) -> ()
                  n294 = local write "Server address"(w543) -> ()
                }
                frame "Default Traverse Name" {
                  n295 = global write "Trav_pos_global.vi" "Default Traverse Setup"(w544) -> ()
                }
                frame "Server port number" {
                  n296 = Decimal String To Number(string=w547) -> (number=w546:i32)  [unwired: 3 out]
                  n297 = To Unsigned Long Integer(number=w546) -> (unsigned 32bit integer=w545:u32)
                  n298 = local write "Server port number"(w545) -> ()
                  n299 = global write "Preference_global.vi" "Server port number"(w545) -> ()
                }
                frame "Analogue Device Serial No." {
                  n300 = local write "Analogue Device Serial No."(w548) -> ()
                }
                frame "PWA Device Serial No." {
                  n301 = local write "PWA Device Serial No."(w549) -> ()
                }
                frame "Default Source Establishment Time (s)" {
                  n302 = Fract/Exp String To Number(string=w551) -> (number=w550:dbl)  [unwired: 4 out]
                  n303 = global write "Preference_global.vi" "Default Source Establishment Time (s)"(w550) -> ()
                  n304 = local write "Default Source Establishment Time (s)"(w550) -> ()
                }
                frame "Tunnel Speed Control" {
                  n305 = Equal?(x="TRUE", y=w553) -> (x = y?=w552:bool)
                  n306 = local write "Tunnel Speed Control"(w552) -> ()
                  n307 = global write "Preference_global.vi" "Tunnel Speed Control"(w552) -> ()
                }
                frame "LabVIEW Administrators" {
                  n308 = call "Get_array_values_fr_String.vi"("String Value"=w556) -> ("String array"=w555:string[])  [unwired: 1 out]
                  n309 = global write "Preference_global.vi" "LabVIEW Administrators"(w555) -> ()
                  n310 = local write "LabVIEW Administrators"(w555) -> ()
                }
                frame "SMTP server IP address" {
                  n311 = local write "SMTP server IP address"(w557) -> ()
                  n312 = global write "Preference_global.vi" "SMTP server IP address"(w557) -> ()
                }
                frame "Server Comms" {
                  n313 = Equal?(x="TRUE", y=w560) -> (x = y?=w559:bool)
                  n314 = case shown="False" w559 {
                    tunnel: [Server_Comms."Do Not Link To Server" ("Server Comms") Server_Comms."Server Link Healthy" ("Server Comms")] -> w558
                    frame False {
                    }
                    frame True {
                    }
                  }
                  n315 = local write "Server Comms"(w558) -> ()
                  n316 = global write "Preference_global.vi" "Server Comms"(w558) -> ()
                }
                frame "Temperature" {
                  n317 = global write "Preference_global.vi" "Temperature"(w564) -> ()
                  n318 = local write "Temperature"(w564) -> ()
                }
                frame "Abs Press (mbar)" {
                  n319 = global write "Preference_global.vi" "Abs Press (mbar)"(w565) -> ()
                  n320 = local write "Abs Press (mbar)"(w565) -> ()
                }
                frame "Qnet Site Root" {
                  n321 = String To Path(string=w567) -> (path=w566:path)
                  n322 = global write "Qnet_Globals.vi" "Local Site Root"(w566) -> ()
                  n323 = local write "Qnet Site Root"(w566) -> ()
                }
                frame "Current Overhead Factor" {
                  n324 = Fract/Exp String To Number(string=w569) -> (number=w568:dbl)  [unwired: 4 out]
                  n325 = call "Overhead_Factor.vi"("Current Overhead Factor In"=w568, "Mode"=Overhead."Initialise totals to 3hr") -> ()  [unwired: 2 in, 1 out]
                }
                frame "Auto Calib Error fr Previous" {
                  n326 = Fract/Exp String To Number(string=w572) -> (number=w571:dbl)  [unwired: 4 out]
                  n327 = global write "Preference_global.vi" "% Error From Previous Calib"(w571) -> ()
                  n328 = local write "% Error From Previous Calib"(w571) -> ()
                }
                frame "Auto Calib Error fr First" {
                  n329 = Fract/Exp String To Number(string=w574) -> (number=w573:dbl)  [unwired: 4 out]
                  n330 = global write "Preference_global.vi" "% Error From First Calib"(w573) -> ()
                  n331 = local write "% Error From First Calib"(w573) -> ()
                }
              }
            }
            frame "Char not in string" {
            }
          }
        }
        n332 = local read "Post Processing Machine"() -> (w525:bool)
        n333 = Select(t="Check file permission status", s=w525, f="is traverse setup blank?") -> (s? t:f=w523:string)
        n334 = Build Array (concatenate)(w528, w526) -> (w527:path[])
      }
      frame "is traverse setup blank?" {
        n335 = local read "Data Folder"() -> (w581:path)
        n336 = global read "Trav_pos_global.vi" "Default Traverse Setup"() -> (w575:string)
        n337 = Build Path(base path=w581, name or relative path="Preferences") -> (appended path=w580:path)
        n338 = Build Path(base path=w580, name or relative path=w584) -> (appended path=w579:path)
        n339 = List Folder(path=w579) -> (folder names=w577:string[])  [unwired: 1 in, 5 out]
        n340 = Search 1D Array(1D array=w577, element=w575) -> (index of element=w578:i32)  [unwired: 1 out]
        n341 = case shown="0, Default" w578 {
          tunnel: w577 -> [_ w590]
          tunnel: [w588 w589] -> w576
          tunnel: w575 -> [w588 _]
          frame 0, Default {
          }
          frame -1 {
            n342 = Index Array(array=w590, index=0) -> (element=w589:string)
          }
        }
        n343 = global write "Trav_pos_global.vi" "Default Traverse Setup"(w576) -> ()
      }
      frame "Please Enter new  Traverse Setup" {
        n344 = global read "Trav_pos_global.vi" "Default Traverse Setup"() -> (w594:string)
        n345 = String Length(string=w594) -> (length=w599:i32)
        n346 = In Range and Coerce(upper limit=w596, x=w599, lower limit=w597) -> (In Range?=w595:bool)  [unwired: 1 out]
        n347 = case shown="False" w595 {
          tunnel: w594 -> [w610 w618]
          tunnel: ["Please Enter new  Traverse Setup" "Update Traverse setup menu ring"] -> w598
          tunnel: [w603 w618] -> w593
          tunnel: w597 -> [w607 _]
          tunnel: w596 -> [w606 _]
          frame False {
            n348 = Format Into String(format string="Please Enter a Traverse Setup Name\nIt must be between %d and %d Characters" ("Message to user"), w607, w606) -> (resulting string=w605:string)  [unwired: 2 in, 1 out]
            n349 = call "Input_String_Dialog.vi"("Value"=w610, "Message to user"=w605) -> ("Ok Out"=w602:bool, "Output string"=w604:string)
            n350 = case shown="False" w602 {
              tunnel: w604 -> [_ w615]
              tunnel: [w611 w614] -> w603
              frame False {
                n351 = property on="Default Traverse Name" class="Ring (strict)"() -> ("Strings []"=w612:string[])  [unwired: 2 in, 2 out]
                n352 = Index Array(array=w612, index=0) -> (element=w611:string)
              }
              frame True {
                n353 = call "Fast_string_Replace.vi"("Replace match with:"="_", "Input String"=w615, "regular expression"=" ") -> ("Output String"=w614:string)  [unwired: 2 out]
              }
            }
          }
          frame True {
          }
        }
        n354 = global write "Trav_pos_global.vi" "Default Traverse Setup"(w593) -> ()
      }
      frame "Update Traverse setup menu ring" {
        n355 = global read "Trav_pos_global.vi" "Default Traverse Setup"() -> (w623:string)
        n356 = local read "Data Folder"() -> (w629:path)
        n357 = Build Path(base path=w629, name or relative path="Preferences") -> (appended path=w628:path)
        n358 = Build Path(base path=w628, name or relative path=w621) -> (appended path=w627:path)
        n359 = List Folder(path=w627) -> (folder names=w625:string[])  [unwired: 1 in, 5 out]
        n360 = Build Array (concatenate)(w625, "--New Traverse Setup--") -> (w624:string[])
        n361 = Search 1D Array(1D array=w624, element=w623) -> (index of element=w631:i32)  [unwired: 1 out]
        n362 = case shown="-1" w631 {
          tunnel: [w637 0] -> w633
          tunnel: w624 -> [w636 w640]
          tunnel: w623 -> [_ w639]
          tunnel: w631 -> [w637 _]
          tunnel: [w636 w638] -> w622
          frame 0, Default {
          }
          frame -1 {
            n363 = Build Array (concatenate)(w639, w640) -> (w638:string[])
          }
        }
        n364 = local write "Default Traverse Name"(w633) -> ()
        n365 = property on="Default Traverse Name" class="Ring (strict)"("Strings []"=w622) -> ()  [unwired: 2 in, 2 out]
      }
      frame "Create Traverse setup" {
        n366 = local read "Templates"() -> (w643:path)
        n367 = Build Path(base path=w643, name or relative path="All_Traverses") -> (appended path=w649:path)
        n368 = stacked-sequence {
          seq-local: [w654 _] -> [_ w682]
          seq-local: [w653 _] -> [_ _]
          tunnel: w649 -> [w656 _]
          tunnel: [w659 _] -> w646
          tunnel: [w658 _] -> w645
          tunnel: w643 -> [_ w681]
          tunnel: [_ w679] -> w642
          frame #0 {
            w662 = "Default_Space_file.xls" ("name or relative path")
            w657 = "Traverse_Setup.xls" ("name or relative path")
            n369 = global read "Trav_pos_global.vi" "Default Traverse Setup"() -> (w653:string)
            n370 = global read "Constants_global.vi" "Traverse folder"() -> (w666:path)
            n371 = Build Path(base path=w656, name or relative path=w662) -> (appended path=w660:path)
            n372 = Build Path(base path=w656, name or relative path=w657) -> (appended path=w655:path)
            n373 = Build Path(base path=w666, name or relative path=w653) -> (appended path=w654:path)
            n374 = Build Path(base path=w654, name or relative path="Trav_Space_Files") -> (appended path=w663:path)
            n375 = Build Path(base path=w663, name or relative path=w662) -> (appended path=w659:path)
            n376 = call "Does_file_exist_(simple).vi"("Pathname"=w659) -> ("exists?"=w661:bool)
            n377 = case shown="False" w661 {
              tunnel: w660 -> [w669 _]
              tunnel: w659 -> [w668 _]
              frame False {
                n378 = call "Create_directory_path.vi"("Path name"=w668) -> ("Path name Out"=w667:path)
                n379 = Copy(10:w667, 11:w669) -> ()  [unwired: 1 in, 5 out]
              }
              frame True {
              }
            }
            n380 = Build Path(base path=w654, name or relative path=w657) -> (appended path=w658:path)
            n381 = call "Does_file_exist_(simple).vi"("Pathname"=w658) -> ("exists?"=w665:bool)
            n382 = case shown="False" w665 {
              tunnel: w655 -> [w678 _]
              tunnel: w658 -> [w674 _]
              tunnel: w653 -> [w677 _]
              frame False {
                w670 = TRUE  # append to file? (new file:F)
                n383 = call "Create_directory_path.vi"("Path name"=w674) -> ("Path name Out"=w673:path)
                n384 = call "Read_File_Simple.vi"("Filename"=w678) -> ("string"=w676:string)  [unwired: 2 in, 7 out]
                n385 = call "Fast_string_Replace.vi"("Replace match with:"=w677, "Input String"=w676, "regular expression"="A_Tunnel") -> ("Output String"=w672:string)  [unwired: 2 out]
                n386 = call "Write_Characters_To_File.vi"("file path (dialog if empty)"=w673, "advisory dialog? (display:T)"=TRUE, "character string"=w672, "append to file? (new file:F)"=w670) -> ()  [unwired: 1 in, 4 out]
              }
              frame True {
              }
            }
          }
          frame #1 {
            w680 = "Traverse_Preferences.txt" ("name or relative path")
            n387 = Build Path(base path=w682, name or relative path=w680) -> (appended path=w679:path)
            n388 = Build Path(base path=w681, name or relative path=w680) -> (appended path=w683:path)
            n389 = call "Does_file_exist_(simple).vi"("Pathname"=w679) -> ("exists?"=w684:bool)
            n390 = case shown="False" w684 {
              tunnel: w683 -> [w687 _]
              tunnel: w679 -> [w686 _]
              frame False {
                n391 = call "Create_directory_path.vi"("Path name"=w686) -> ("Path name Out"=w685:path)
                n392 = Copy(10:w685, 11:w687) -> ()  [unwired: 1 in, 5 out]
              }
              frame True {
              }
            }
          }
        }
        n393 = Build Array (concatenate)(w648, w645, w642, w646) -> (w647:path[])
      }
      frame "Check file permission status" {
        n394 = for {
          tunnel: w692 -> [w706] mode=indexing
          shift-right: [w703] -> w689
          shift-left: "" -> [w704]
          n395 = call "Can_File_be_Editted.vi"("Filename"=w706) -> ("File Permissions OK?"=w707:bool, "Comment String"=w705:string)  [unwired: 2 out]
          n396 = case shown="False" w707 {
            tunnel: w706 -> [w712 _]
            tunnel: w705 -> [w711 _]
            tunnel: w704 -> [w710 w713]
            tunnel: [w709 w713] -> w703
            frame False {
              n397 = Format Into String(format string="\"%s\" %s\n", initial string=w710, w712, w711) -> (resulting string=w709:string)  [unwired: 1 in, 1 out]
            }
            frame True {
            }
          }
        }
        n398 = case shown="\"Load, Edit then Save\"" w693 {
          tunnel: ["Output Dev Number" w715 "Output Dev Number"] -> w694
          frame "Save Preferences to file" {
          }
          frame "Load, Edit then Save" {
            n399 = local read "Post Processing Machine"() -> (w718:bool)
            n400 = Select(t="Data Folder Changed?", s=w718, f="What next1") -> (s? t:f=w715:string)
          }
          frame "Load Preferences from file" {
          }
        }
        n401 = Empty String/Path?(string/path=w689) -> (empty?=w690:bool)
        n402 = case shown="True" w690 {
          tunnel: w689 -> [w702 _]
          frame False {
            n403 = Concatenate Strings("The following file permissions need to be sorted out before the software will run correctly.\n\n" ("string"), w702) -> (w700:string)
            n404 = Two Button Dialog(message=w700, 1:"Continue" ("F button name (\"Cancel\")"), 2:"Abort" ("F button name (\"Cancel\")")) -> (T button?=w697:bool)
            n405 = Stop(stop? (T)=w697) -> ()
          }
          frame True {
          }
        }
      }
      frame "What next1" {
        n406 = property on="Rig Setup" class="Ring (strict)"() -> ("Strings []"=w722:string[])  [unwired: 2 in, 2 out]
        n407 = Array Size(array=w722) -> (size(s)=w726:i32)
        n408 = Decrement(x=w726) -> (x-1=w725:i32)
        n409 = Equal?(x=w725, y="Rig Setup") -> (x = y?=w724:bool)
        n410 = case shown="False" w724 {
          tunnel: [w730 "Please Enter New Rig Name" ("t")] -> w723
          tunnel: w722 -> [w733 _]
          tunnel: "Rig Setup" -> [w732 _]
          frame False {
            n411 = global read "Preference_global.vi" "Rig Setup"() -> (w734:string)
            n412 = Index Array(array=w733, index=w732) -> (element=w729:string)
            n413 = Not Equal?(x=w729, y=w734) -> (x != y?=w731:bool)
            n414 = case shown="False" w731 {
              tunnel: ["What next2" ("f") "Update Rig setup menu ring" ("t")] -> w730
              tunnel: w729 -> [_ w736]
              frame False {
              }
              frame True {
                n415 = global write "Preference_global.vi" "Rig Setup"(w736) -> ()
              }
            }
          }
          frame True {
            n416 = global write "Preference_global.vi" "Rig Setup"("") -> ()
          }
        }
      }
      frame "What next2" {
        n417 = property on="Default Traverse Name" class="Ring (strict)"() -> ("Strings []"=w742:string[])  [unwired: 2 in, 2 out]
        n418 = Array Size(array=w742) -> (size(s)=w746:i32)
        n419 = Decrement(x=w746) -> (x-1=w745:i32)
        n420 = Equal?(x=w745, y="Default Traverse Name") -> (x = y?=w744:bool)
        n421 = case shown="False" w744 {
          tunnel: [w750 "Please Enter new  Traverse Setup" ("t")] -> w743
          tunnel: w742 -> [w754 _]
          tunnel: "Default Traverse Name" -> [w753 _]
          frame False {
            n422 = global read "Trav_pos_global.vi" "Default Traverse Setup"() -> (w752:string)
            n423 = Index Array(array=w754, index=w753) -> (element=w749:string)
            n424 = Not Equal?(x=w749, y=w752) -> (x != y?=w751:bool)
            n425 = case shown="False" w751 {
              tunnel: ["Data Folder Changed?" ("f") "Update Traverse setup menu ring" ("t")] -> w750
              tunnel: w749 -> [_ w756]
              frame False {
              }
              frame True {
                n426 = global write "Trav_pos_global.vi" "Default Traverse Setup"(w756) -> ()
              }
            }
          }
          frame True {
            n427 = global write "Trav_pos_global.vi" "Default Traverse Setup"("") -> ()
          }
        }
      }
      frame "Data Folder Changed?" {
        w761 = "Please Select your data folder"
        n428 = global read "Constants_global.vi" "Data Folder"() -> (w768:path)
        n429 = local read "Data Folder"() -> (w769:path)
        n430 = property on="OK" class="Bool (strict)"("Visible"=TRUE) -> ()  [unwired: 2 in, 2 out]
        n431 = while {
          shift-right: [w778] -> _
          shift-left: _ -> [w777]
          tunnel: [w776] -> w763
          stop <- TRUE stop-if-true
          n432 = local read "Post Processing Machine"() -> (w778:bool)
          n433 = Not Equal?(x=w778, y=w777) -> (x != y?=w776:bool)
        }
        n434 = Not Equal?(x=w768, y=w769) -> (x != y?=w767:bool)
        n435 = Select(t=w761, s=w767, f="Has OK has been pressed?") -> (s? t:f=w760:string)
        n436 = case shown="True" w763 {
          tunnel: [w772 w774] -> w762
          tunnel: w761 -> [_ w774]
          tunnel: w760 -> [w772 _]
          frame False {
          }
          frame True {
            n437 = global write "Preference_global.vi" "Rig Setup"("") -> ()
          }
        }
      }
      frame "Has OK has been pressed?" {
        n438 = flat-sequence {
          tunnel: ["OK"] -> w780
          frame #0 {
            n439 = Wait (ms)(milliseconds to wait=u32 100) -> ()  [unwired: 1 out]
          }
          frame #1 {
          }
        }
        n440 = local read "Post Processing Machine"() -> (w781:bool)
        n441 = case shown="False" w780 {
          tunnel: w781 -> [w786 w792]
          tunnel: [w785 w789] -> w779
          frame False {
            n442 = Select(t="Data Folder Changed?", s=w786, f="What next1") -> (s? t:f=w785:string)
          }
          frame True {
            n443 = Select(t="Save Preference File", s=w792, f="Output Dev Number") -> (s? t:f=w789:string)
          }
        }
      }
      frame "Output Dev Number" {
        n444 = stacked-sequence {
          seq-local: [w800 _ _] -> [_ w836 _]
          tunnel: w797 -> [_ _ _]
          frame #0 {
            w803 = T8 0 items=["Canonical Names Only"=0, "Aliases Only"=1, "Include Matching Aliases"=2, "Include All Aliases"=4] ("Search Mode")
            n445 = VISA Find Resource(10:w803) -> (3:w802:string[])  [unwired: 1 in, 3 out]
            n446 = for {
              shift-right: [w818] -> w800
              shift-left: string[] [] -> [w819]
              tunnel: w802 -> [w808] mode=indexing
              n447 = Reverse String(1:w808) -> (0:w816:string)
              n448 = Match Pattern(string=w816, regular expression="::") -> (before substring=w815:string)  [unwired: 4 out]
              n449 = Match Pattern(string=w808, regular expression="NI-VISA") -> (offset past match=w807:i32)  [unwired: 4 out]
              n450 = Reverse String(1:w815) -> (0:w813:string)
              n451 = Less Than 0?(x=w807) -> (x < 0?=w805:bool)
              n452 = Equal?(x=w813, y="INSTR") -> (x = y?=w811:bool)
              n453 = Equal?(x=w813, y="RAW") -> (x = y?=w810:bool)
              n454 = Or(x=w811, y=w810) -> (x .or. y?=w806:bool)
              n455 = And(x=w806, y=w805) -> (x .and. y?=w804:bool)
              n456 = case shown="True" w804 {
                tunnel: w819 -> [w820 w823]
                tunnel: [w820 w822] -> w818
                tunnel: w808 -> [_ w821]
                frame False {
                }
                frame True {
                  n457 = Build Array (concatenate)(w823, w821) -> (w822:string[])
                }
              }
            }
          }
          frame #1 {
            w828 = "Dev" ("format string")
            n458 = local read "Analogue Device Serial No."() -> (w832:string)
            n459 = String Length(string=w828) -> (length=w830:i32)
            n460 = local read "PWA Device Serial No."() -> (w826:string)
            n461 = String Subset(string=w832, length (rest)=w830) -> (substring=w834:string)  [unwired: 1 out]
            n462 = String Subset(string=w826, length (rest)=w830) -> (substring=w829:string)  [unwired: 1 out]
            n463 = Equal?(x=w834, y=w828) -> (x = y?=w831:bool)
            n464 = Equal?(x=w828, y=w829) -> (x = y?=w827:bool)
            n465 = for {
              tunnel: w832 -> [w855]
              tunnel: w836 -> [w853] mode=indexing
              tunnel: [w854] -> w848 mode=indexing
              tunnel: w826 -> [w852]
              tunnel: [w851] -> w845 mode=indexing
              n466 = Match Pattern(string=w853, regular expression=w855) -> (offset past match=w854:i32)  [unwired: 1 in, 3 out]
              n467 = Match Pattern(string=w853, regular expression=w852) -> (offset past match=w851:i32)  [unwired: 1 in, 3 out]
            }
            n468 = Array Max & Min(array=w848) -> (max index (indices)=w849:i32)  [unwired: 3 out]
            n469 = Array Max & Min(array=w845) -> (max index (indices)=w847:i32)  [unwired: 3 out]
            n470 = Increment(x=w847) -> (x+1=w838:i32)
            n471 = Increment(x=w849) -> (x+1=w842:i32)
            n472 = Equal To 0?(x=w842) -> (x = 0?=w844:bool)
            n473 = Equal To 0?(x=w838) -> (x = 0?=w839:bool)
            n474 = Select(t=1, s=w844, f=w842) -> (s? t:f=w843:i32)
            n475 = Select(t=1, s=w839, f=w838) -> (s? t:f=w837:i32)
            n476 = Format Into String(format string="Dev%d", w843) -> (resulting string=w833:string)  [unwired: 2 in, 1 out]
            n477 = Format Into String(format string="Dev%d", w837) -> (resulting string=w825:string)  [unwired: 2 in, 1 out]
            n478 = Select(t=w832, s=w831, f=w833) -> (s? t:f=w835:string)
            n479 = Select(t=w826, s=w827, f=w825) -> (s? t:f=w824:string)
            n480 = global write "PWAtasksGLOBAL.vi" "Analogue Dev Name"(w835) -> ()
            n481 = global write "PWAtasksGLOBAL.vi" "PWA Dev Name"(w824) -> ()
          }
          frame #2 {
            n482 = for {
              tunnel: string[] ["Raw_Calibrations", "Raw_Measurements", "Results", "Calibrations", "Commands"] -> [w860] mode=indexing
              n483 = call "Data_folder_Path.vi"("Data Type"=w860) -> ("Data Folder"=w859:path)  [unwired: 1 in]
              n484 = Build Path(base path=w859, name or relative path="Test" ("Substring")) -> (appended path=w862:path)
              n485 = call "Create_directory_path.vi"("Path name"=w862) -> ()  [unwired: 1 out]
            }
            n486 = call "Data_folder_Path.vi"("Data Type"="Results_Post_Processed" ("element")) -> ("Data Folder"=w856:path)  [unwired: 1 in]
            n487 = call "Create_directory_path.vi"("Path name"=w856) -> ()  [unwired: 1 out]
          }
        }
      }
      frame "Save Preference File" {
        n488 = global read "Constants_global.vi" "General folder"() -> (w866:path)
        n489 = call "Date_and_Time_to_string.vi"() -> ("Date and time (spreadsheet)"=w874:string)
        n490 = Build Path(base path=w866, name or relative path=w865) -> (appended path=w864:path)
        n491 = for {
          tunnel: w873 -> [w884] mode=indexing
          shift-right: [w880] -> w872
          shift-left: w874 -> [w882]
          n492 = case shown="\"Analogue Device Serial No.\"" w884 {
            tunnel: w884 -> [w887 _ _ _ _ _ _ _ _ _ _ _ _ _ _ _ _]
            tunnel: ["No Match" "Server address" w890 w892 w894 w898 "SMTP server IP address" "PWA Device Serial No." "Analogue Device Serial No." w902 w904 "Temperature" "Abs Press (mbar)" w909 w914 w917 w920] -> w883
            frame "No Match", Default {
              n493 = call "Was_string_matched.vi"("Match Error"=TRUE, "Variable name"=w887) -> ()  [unwired: 1 in]
            }
            frame "Server address" {
              n494 = global write "Preference_global.vi" "Server address"("Server address") -> ()
            }
            frame "Server port number" {
              n495 = global write "Preference_global.vi" "Server port number"("Server port number") -> ()
              n496 = Number To Decimal String(number="Server port number") -> (decimal integer string=w890:string)  [unwired: 1 out]
            }
            frame "Default Source Establishment Time (s)" {
              n497 = global write "Preference_global.vi" "Default Source Establishment Time (s)"("Default Source Establishment Time (s)") -> ()
              n498 = Number To Decimal String(number="Default Source Establishment Time (s)") -> (decimal integer string=w892:string)  [unwired: 1 out]
            }
            frame "Tunnel Speed Control" {
              n499 = global write "Preference_global.vi" "Tunnel Speed Control"("Tunnel Speed Control") -> ()
              n500 = Select(t="TRUE", s="Tunnel Speed Control", f="FALSE") -> (s? t:f=w894:string)
            }
            frame "LabVIEW Administrators" {
              n501 = global write "Preference_global.vi" "LabVIEW Administrators"("LabVIEW Administrators") -> ()
              n502 = call "Put_Array_into_String.vi"("String array"="LabVIEW Administrators") -> ("String Value"=w898:string)
            }
            frame "SMTP server IP address" {
              n503 = global write "Preference_global.vi" "SMTP server IP address"("SMTP server IP address") -> ()
            }
            frame "PWA Device Serial No." {
            }
            frame "Analogue Device Serial No." {
            }
            frame "Default Traverse Name" {
              n504 = global read "Trav_pos_global.vi" "Default Traverse Setup"() -> (w902:string)
            }
            frame "Server Comms" {
              n505 = case shown="\"Server Link Healthy\"" "Server Comms" {
                tunnel: ["TRUE" "FALSE"] -> w904
                frame "Server Link Healthy" {
                }
                frame "Do Not Link To Server" {
                }
              }
              n506 = global write "Preference_global.vi" "Server Comms"("Server Comms") -> ()
            }
            frame "Temperature" {
              n507 = global write "Preference_global.vi" "Temperature"("Temperature") -> ()
            }
            frame "Abs Press (mbar)" {
              n508 = global write "Preference_global.vi" "Abs Press (mbar)"("Abs Press (mbar)") -> ()
            }
            frame "Current Overhead Factor" {
              n509 = call "Overhead_Factor.vi"("Mode"=Overhead."Read Current Overhead") -> ("Current Overhead Factor"=w911:dbl)  [unwired: 3 in]
              n510 = Number To Fractional String(number=w911, precision (6)=i16 4) -> (F-format string=w909:string)  [unwired: 2 out]
            }
            frame "Auto Calib Error fr Previous" {
              n511 = global write "Preference_global.vi" "% Error From Previous Calib"("% Error From Previous Calib") -> ()
              n512 = Number To Fractional String(number="% Error From Previous Calib", precision (6)=i16 2) -> (F-format string=w914:string)  [unwired: 2 out]
            }
            frame "Auto Calib Error fr First" {
              n513 = global write "Preference_global.vi" "% Error From First Calib"("% Error From First Calib") -> ()
              n514 = Number To Fractional String(number="% Error From First Calib", precision (6)=i16 2) -> (F-format string=w917:string)  [unwired: 2 out]
            }
            frame "Qnet Site Root" {
              n515 = global write "Qnet_Globals.vi" "Local Site Root"("Qnet Site Root") -> ()
              n516 = Path To String(path="Qnet Site Root") -> (string=w920:string)
            }
          }
          n517 = call "Characters_to_string.vi"("Characters to write"=w883, "Label for characters"=w884) -> ("Output string"=w881:string)
          n518 = Concatenate Strings(w882, w881) -> (w880:string)
        }
        n519 = case shown="\"Load, Edit then Save\"" w868 {
          tunnel: [TRUE TRUE TRUE] -> w867
          frame "Load, Edit then Save" {
            n520 = Current VI's Path() -> (path=w876:path)
            n521 = call "Open_Close_Front_Panel.ph.vi"("Front Panel Window:Open"=FALSE, "VI path"=w876) -> ()  [unwired: 2 out]
          }
          frame "Load Preferences from file" {
          }
          frame "Save Preferences to file" {
          }
        }
        n522 = call "Write_Characters_To_File.vi"("file path (dialog if empty)"=w864, "advisory dialog? (display:T)"=FALSE, "character string"=w872, "append to file? (new file:F)"=FALSE) -> ()  [unwired: 1 in, 4 out]
      }
      frame "Save SW Preferences" {
        w936 = FALSE  # append to file? (new file:F)
        w937 = FALSE  # advisory dialog? (display:T)
        n523 = local read "Post Processing Machine"() -> (w926:bool)
        n524 = Path To String(path="Data Folder") -> (string=w928:string)
        n525 = global read "Preference_global.vi" "Server Comms"() -> (w932:T2)
        n526 = call "Characters_to_string.vi"("Characters to write"=w928, "Label for characters"=w930) -> ("Output string"=w938:string)
        n527 = Select(t="True", s=w926, f="False") -> (s? t:f=w923:string)
        n528 = call "Characters_to_string.vi"("Characters to write"=w923, "Label for characters"=w921) -> ("Output string"=w922:string)
        n529 = call "Date_and_Time_to_string.vi"() -> ("Date and time (spreadsheet)"=w933:string)
        n530 = case shown="\"Server Link Healthy\"" w932 {
          tunnel: ["Update Served VI file" "Update Local Adam Table"] -> w931
          frame "Server Link Healthy" {
          }
          frame "Do Not Link To Server" {
          }
        }
        n531 = Concatenate Strings(w933, w938, w922) -> (w934:string)
        n532 = local read "EnFlo SW Preferences"() -> (w935:path)
        n533 = call "Write_Characters_To_File.vi"("file path (dialog if empty)"=w935, "advisory dialog? (display:T)"=w937, "character string"=w934, "append to file? (new file:F)"=w936) -> ()  [unwired: 1 in, 4 out]
      }
      frame "Update Local Adam Table" {
        n534 = stacked-sequence {
          seq-local: [w952 _] -> [_ w966]
          tunnel: ["Update Served VI file" _] -> w944
          frame #0 {
            w952 = T9 {"Ch Name"="", "Type"=enum."4011", "Function"=enum."Analogue Input", "Ch State"=enum."On", "Calibration type"=enum."Raw", "A"=0.0, "B"=0.0, "C"=0.0, "D"=0.0, "Comments"="", "Address"={"Main"=0, "Ch."=0, "Sub"=0, "Port Name"=""}, "String"="", "Duty"=0} ("Ch Discription")
            n535 = global read "Preference_global.vi" "Abs Press (mbar)"() -> (w949:string)
            n536 = global read "Preference_global.vi" "Temperature"() -> (w950:string)
            n537 = Bundle By Name(cluster=w952, "Type"=Module_type_ADAM."Hold Value", "Calibration type"=Calib_type_ADAM."Raw", "A"=1.0) -> (w953:T9)
            n538 = Build Array(w950, w949) -> (w948:string[])
            n539 = for {
              tunnel: [w959] -> w951 mode=indexing
              tunnel: w953 -> [w958]
              tunnel: w948 -> [w957] mode=indexing
              n540 = Bundle By Name(cluster=w958, "Ch Name"=w957) -> (w959:T9)
            }
            n541 = call "Update_Ch_Discription_client.vi"("Channels to update In"=w951) -> ()  [unwired: 1 out]
          }
          frame #1 {
            n542 = global read "Preference_global.vi" "Rig Setup"() -> (w961:string)
            n543 = call "Get_Current_Scan_client.vi"() -> ("Ch Description Array"=w967:T9[])  [unwired: 1 in, 3 out]
            n544 = Match Pattern(string=w961, regular expression="-") -> (before substring=w960:string)  [unwired: 4 out]
            n545 = Format Into String(format string="%s Metadata:" ("Format String"), w960) -> (resulting string=w969:string)  [unwired: 2 in, 1 out]
            n546 = Initialize Array(w966, 0 ("dimension size")) -> (w964:T9[])
            n547 = for {
              shift-right: [w980] -> w963
              shift-left: w964 -> [w981]
              tunnel: w967 -> [w972] mode=indexing
              tunnel: w969 -> [w979]
              tunnel: "Metadata:" ("Format String") -> [w978]
              n548 = Unbundle By Name(w972) -> ("Ch Name"=w971:string)
              n549 = Match Pattern(string=w971, regular expression=w979) -> (offset past match=w976:i32)  [unwired: 4 out]
              n550 = Match Pattern(string=w971, regular expression=w978) -> (offset past match=w977:i32)  [unwired: 4 out]
              n551 = Greater Or Equal To 0?(x=w977) -> (x >= 0?=w974:bool)
              n552 = Less Than 0?(x=w976) -> (x < 0?=w975:bool)
              n553 = And(x=w975, y=w974) -> (x .and. y?=w973:bool)
              n554 = case shown="True" w973 {
                tunnel: w981 -> [w982 w987]
                tunnel: [w982 w986] -> w980
                tunnel: w972 -> [_ w985]
                frame False {
                }
                frame True {
                  n555 = Bundle By Name(cluster=w985, "Ch State"=Channel_State."Off") -> (w983:T9)
                  n556 = Build Array (concatenate)(w987, w983) -> (w986:T9[])
                }
              }
            }
            n557 = call "Update_Ch_Discription_client.vi"("Channels to update In"=w963) -> ()  [unwired: 1 out]
          }
        }
      }
      frame "Update Served VI file" {
        # "Template"
        # "Orig"
        n558 = global read "Constants_global.vi" "General folder"() -> (w996:path)
        n559 = Build Path(base path=w996, name or relative path=w989) -> (appended path=w991:path)
        n560 = Build Array("Served:VI:Name", "Served:VI:Path", "Server:IP Number:& Port No") -> (w993:string[])
        n561 = stacked-sequence {
          seq-local: [w999 _ _ _] -> [_ _ w1009 _]
          seq-local: [_ w1006 _ _] -> [_ _ w1010 _]
          seq-local: [_ _ w1011 _] -> [_ _ _ w1036]
          tunnel: w993 -> [w1001 w1007 _ w1037]
          tunnel: w991 -> [w1000 _ _ w1038]
          tunnel: w989 -> [_ w1003 _ _]
          frame #0 {
            n562 = call "Read_Ch_data_file.vi"("Present Channels"=w1001, "Output"=enum16{"All Ch data", "The last few rows"}."All Ch data", "Filename"=w1000) -> ("Channel Values"=w999:string[][])  [unwired: 2 in, 4 out]
          }
          frame #1 {
            n563 = local read "Templates"() -> (w1005:path)
            n564 = Build Path(base path=w1005, name or relative path=w1003) -> (appended path=w1004:path)
            n565 = call "Read_Ch_data_file.vi"("Present Channels"=w1007, "Output"=enum16{"All Ch data", "The last few rows"}."All Ch data", "Filename"=w1004) -> ("Channel Values"=w1006:string[][])  [unwired: 2 in, 4 out]
          }
          frame #2 {
            n566 = Index Array(array=w1009, index (col)=0 ("Index")) -> (element=w1014:string[])  [unwired: 1 in]
            n567 = To Upper Case(1:w1010) -> (0:w1012:string[][])
            n568 = To Upper Case(1:w1014) -> (0:w1013:string[])
            n569 = for {
              tunnel: w1013 -> [w1017]
              tunnel: w1010 -> [w1022] mode=indexing
              tunnel: w1012 -> [w1016] mode=indexing
              tunnel: [w1019] -> w1011 mode=indexing
              tunnel: w1009 -> [w1018]
              n570 = Index Array(array=w1016, index=0 ("Index")) -> (element=w1020:string)
              n571 = Search 1D Array(1D array=w1017, element=w1020) -> (index of element=w1021:i32)  [unwired: 1 out]
              n572 = case shown="0, Default" w1021 {
                tunnel: w1022 -> [w1031 w1032]
                tunnel: w1021 -> [w1028 _]
                tunnel: [w1024 w1032] -> w1019
                tunnel: w1018 -> [w1029 _]
                frame 0, Default {
                  n573 = Index Array(array=w1029, index (row)=w1028, index (col)=2 ("Index")) -> (element=w1026:string)
                  n574 = Array Subset(array=w1031, length=2) -> (w1025:string[])  [unwired: 1 in]
                  n575 = Build Array (concatenate)(w1025, w1026) -> (w1024:string[])
                }
                frame -1 {
                }
              }
            }
          }
          frame #3 {
            w1033 = FALSE  # Append last row only
            w1034 = FALSE  # Lock File
            w1035 = FALSE  # exists?
            n576 = call "Write_Ch_data_file.vi"("Append last row only"=w1033, "Lock File"=w1034, "exists?"=w1035, "Channel Values"=w1036, "Channel names"=w1037, "Filename"=w1038) -> ()  [unwired: 2 in, 4 out]
          }
        }
      }
      frame "Initialise Globals" {
        w1043 = TRUE  # OK
        w1047 = FALSE  # append to file? (new file:F)
        w1046 = FALSE  # advisory dialog? (display:T)
        n577 = global read "Constants_global.vi" "ADAM setups folder"() -> (w1053:path)
        n578 = global read "Constants_global.vi" "All_Users"() -> (w1042:path)
        n579 = property on="ADAM Setup File" class="Ring (strict)"() -> ("Strings []"=w1048:string[])  [unwired: 2 in, 2 out]
        n580 = Build Path(base path=w1042, name or relative path="Current_Username") -> (appended path=w1040:path)
        n581 = Build Path(base path=w1053, name or relative path="Setup_Files") -> (appended path=w1051:path)
        n582 = global read "Preference_global.vi" "User_Name"() -> (w1039:string)
        n583 = Build Path(base path=w1051, name or relative path="Selected_Filename.txt" ("Substring")) -> (appended path=w1044:path)
        n584 = call "Get_users_email_addresses.vi"("OK"=w1043) -> ()  [unwired: 5 out]
        n585 = Index Array(array=w1048, index="ADAM Setup File") -> (element=w1045:string)
        n586 = call "Write_File_Simple.vi"("character string"=w1039, "file path"=w1040) -> ()  [unwired: 1 in, 2 out]
        n587 = global write "Dynamic_call_global.ph.vi" "Acquisition Interlock"(FALSE ("Acquisition Interlock")) -> ()
        n588 = call "Write_Characters_To_File.vi"("file path (dialog if empty)"=w1044, "advisory dialog? (display:T)"=w1046, "character string"=w1045, "append to file? (new file:F)"=w1047) -> ()  [unwired: 1 in, 4 out]
      }
    }
  }
  n589 = call "Get_IP_Number.vi"() -> ("IP Number"=→"This Machine's IP Number":string)
